vi "Dashboard Main.vi"() -> ()   [LabVIEW 2016]
uses:
  <vilib>/Utility/miscctls.llb/LVRowAndColumnTypeDef.ctl
  <vilib>/event_ctls.llb/eventvkey.ctl
  <vilib>/Rock Robotics/Network Tables/NT Write Boolean.vi
  <vilib>/Rock Robotics/Network Tables/NT Read Numeric Array.vi
  <vilib>/Rock Robotics/WPI/Dashboard/WPI_DashboardLogging Global.vi
  <vilib>/Utility/config.llb/Read Key (Double).vi
  <vilib>/Utility/config.llb/Write Key (Double).vi
  <vilib>/Utility/config.llb/NI_LVConfig.lvlib
panel:
  in  "Camera Settings Right":T1={"Frame Rate"=30, "Compression"=30, "Size"=1, "DB Camera Config"=FALSE} {"Frame Rate" scale=1.0..30.0; "Compression" scale=100.0..-1.0; "Size" items=["640x480", "320x240", "160x120"]}
  in  "Camera Name Right":string(combo)="No Camera Selection"
  out "Camera Info":cluster{"Mbps LED":bool, "Mbps":dbl, "fps":dbl} {"fps" format="%#.1g"; "Mbps" format="%#.1g"}
  in  "Camera Settings":T1={"Frame Rate"=30, "Compression"=30, "Size"=1, "DB Camera Config"=FALSE} {"Frame Rate" scale=1.0..30.0; "Compression" scale=100.0..-1.0; "Size" items=["640x480", "320x240", "160x120"]}
  in  "TCP":refnum<k5>
  in  "Rec Mode":enum32{"Stop", "Record", "Playback"}(radio)
  out "Robot IP":string
  out "Image Message":string="Timeout in Camera Communications"
  in  "Dashboard Tab":T2(tab)
  out "Gear Hopper State":string
  out "Ultrasonic Distance":dbl(slide) scale=0.0..5.0
  in  "Winch Reverse":bool
  in  "Enable PID":bool
  out "Drive Gear":string
  in  "Drive Mode":enum16{"Tank Drive", "Arcade Drive"}(ring)
  in  "Controller Mode":enum16{"X-Box Controller", "Joysticks"}(ring)
  out "Code Version":string
  out "Dashboard Version":string
  in  "Select Auto":string(combo)="Select Autonomous ..."
  out "NT Connection":bool
  out "MotorChart R":cluster{"Numeric":dbl, "Numeric":dbl}(graph)
  out "MotorChart L":cluster{"Numeric":dbl, "Numeric":dbl}(graph)
  out "MotorSliders R":cluster{"MotorSlide1":dbl, "MotorSlide2":dbl} {"MotorSlide2" scale=-1.0..1.0 scale format="%#_2e"; "MotorSlide1" scale=-1.0..1.0 scale format="%#_2e"}
  out "MotorSliders L":cluster{"MotorSlide1":dbl, "MotorSlide2":dbl} {"MotorSlide2" scale=-1.0..1.0 scale format="%#_2e"; "MotorSlide1" scale=-1.0..1.0 scale format="%#_2e"}
  out "Gyro":dbl(knob) scale=0.0..360.0
  out "JS1 Z":dbl(slide) scale=-1.0..1.0 scale format="%#_2e"
  out "JS1 Graph":cluster{"X":dbl, "Y":dbl}[](graph)
  out "JS1 Buttons":T3
  out "JS2 Z":dbl(slide) scale=-1.0..1.0 scale format="%#_2e"
  out "JS2 Graph":cluster{"X":dbl, "Y":dbl}[](graph)
  out "JS2 Buttons":T3
  out "Mode":T4(ring)=enum."Auto Disabled"
  out "Camera Image Right":T5(plugin-control)
  in  "DB/String 9":string
  in  "DB/String 8":string
  in  "DB/String 7":string
  in  "DB/String 6":string
  in  "DB/String 5":string
  in  "DB/String 4":string
  in  "DB/String 3":string
  in  "DB/String 2":string
  in  "DB/String 1":string
  in  "DB/String 0":string
  in  "DB/Slider 0":dbl(slide) scale=0.0..5.0
  in  "DB/Slider 1":dbl(slide) scale=0.0..5.0
  in  "DB/Slider 2":dbl(slide) scale=0.0..5.0
  in  "DB/Slider 3":dbl(slide) scale=0.0..5.0
  out "DB/LED 3":bool
  out "DB/LED 2":bool
  out "DB/LED 1":bool
  out "DB/LED 0":bool
  in  "DB/Button 3":bool
  in  "DB/Button 2":bool
  in  "DB/Button 1":bool
  in  "DB/Button 0":bool caption="New Name"
  in  "High Gear Multiplier":dbl(slide)=1.0 scale=0.0..1.0
  in  "Low Gear Multiplier":dbl(slide)=1.0 scale=0.0..1.0
  out "Robot Status":string
  in  "Ring Light Off":bool
  in  "Ring Light On":bool
  in  "Right Drive Bias":dbl(slide)=1.0 scale=0.9..1.0
  in  "Right Proportional Gain":dbl=0.02
  in  "Left Proportional Gain":dbl=0.02
  in  "Left Drive Bias":dbl(slide)=1.0 scale=0.9..1.0
  in  "Test Slider":dbl(slide) scale=0.0..100.0 scale format="%#_3g"
  in  "On/Off":bool caption="Solenoid"
  in  "Test Name":u16(ring) items=["Select the test to run..."]
  in  "Test Tree":string(tree)
  in  "Motor":cluster{"Value":dbl, "Enable":bool} {"Value" scale=-1.0..1.0 scale format="%#_3g"}
  out "Progress":T6 {"Test Progress" scale=0.0..100.0}
  in  "Rev/Fwd":cluster{"Forward":bool, "Reverse":bool}
  in  "Test Ring":u16(ring) items=["Monochrome", "Color"]
  out "Cmd Status":string
  in  "Execute Command":bool
  in  "Command Params":string[][](table)
  in  "Command Selection":i32(listbox)
  in  "CheckList":i32(listbox)
  out "Tree":string(tree)
  out "Camera Image":T5(plugin-control)
  out "Background":bool
  in  "Camera Name":string(combo)="No Camera Selection"
  # "HW"
  # "HW"
  # "Joysticks"
  # "Ultrasonic Distance"
  # "Drive Motors"
  # "Winch Reverse"
  # "Enable PID"
  # "Front"
  # "0.5"
  # "5"
  # "Controller Mode"
  # "Robot Code Version"
  # "Right"
  # "Left"
  # "Drive Mode"
  # "Dashboard Code Version"
  # "Back"
  # "This tab is a great place for autonomous settings and robot-specific values.\nPlace controls and indicators inside this tab and match name to\nDashboard Variables on robot. You can also delete this comment."
  # "Ring Light On"
  # "Left Drive Bias"
  # "Left Controller Gain"
  # "Right Controller Gain"
  # "Ring Light Off"
  # "Right Drive Bias"
  # "Robot Status"
  # "Low Gear Multiplier"
  # "High Gear Multiplier"
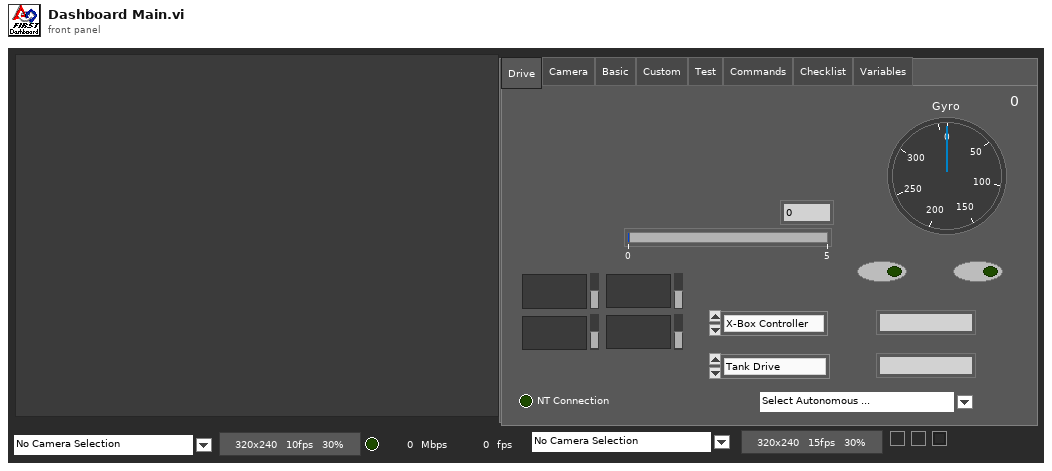
[diagram p1: front panel]
types:
  T1 = cluster{"Frame Rate":i32, "Compression":i32, "Size":u16, "DB Camera Config":bool}
  T2 = enum32{"Drive", "Camera", "Basic", "Custom", "Test", "Commands", "Checklist", "Variables"}
  T3 = cluster{bool, bool, bool, bool, bool, bool, bool, bool, bool, bool, bool, bool}
  T4 = enum8{"Tele-Op Disabled", "Tele-Op Enabled", "Auto Disabled", "Auto Enabled", "Test Disabled", "Test Enabled", "Disconnected", "No Code", "E-Stop"}
  T5 = typedef "IMAQ Image.ctl" = refnum<image>
  T6 = cluster{"Test Progress":u8, "Test Progress Text":string}
  T7 = typedef "Image Type" = u32
  T8 = cluster{"IDs":cluster{"RPC field ID":u16, "Unique ID":u16}, "String":string}
  T9 = enum32{"Drive", "Basic", "Custom", "Test", "Checklist", "Variables"}
  T10 = typedef "NI_LVConfig.lvlib/Config Data RefNum.ctl" = refnum<k1>
  T11 = cluster{"Camera Image":refnum<vi>, "Dashboard Tab":refnum<vi>, "Background":refnum<vi>, "Rec Mode":refnum<vi>, "Test Slider":refnum<vi>, "On/Off ":refnum<vi>, "Test Ring":refnum<vi>, "Rev/Fwd":refnum<vi>, "Test Name":refnum<vi>, "Motor":refnum<vi>, "Progress":refnum<vi>, "CheckList":refnum<vi>, "Tree":refnum<vi>, "Test Tree":refnum<vi>, "Command Params":refnum<vi>, "Command Selection":refnum<vi>, "Execute Command":refnum<vi>, "Cmd Status":refnum<vi>, "Camera Settings":refnum<vi>, "Camera Name":refnum<vi>, "Camera Info":refnum<vi>, "Camera Settings Right":refnum<vi>, "Camera Name Right":refnum<vi>, "Camera Image Right":refnum<vi>}
  T12 = cluster{"Measurement Parameter":i32, "Range Lower Value":dbl, "Range Upper Value":dbl, "Range":bool, "Measurement Type":bool}[]
  T13 = cluster{"Global Rectangle":cluster{"x1Left":i32, "y1Top":i32, "x2Right":i32, "y2Bottom":i32}, "Centroid":cluster{"x":sgl, "y":sgl}, "Object Size":u32, "Score":dbl}[]
  T14 = cluster{"Current Position":enum16{"Closed", "Open"}, "Current State":enum16{"Closed", "Shifting", "Open"}}
  T15 = cluster{"Current Gear":enum16{"Low", "High"}, "Gear Shift State":enum16{"Low", "Shifting", "High"}}
  T16 = cluster{"Error Strings":string, "Disable Counts":cluster{u16, u16}, "Rail Faults":cluster{u16, u16, u16}, "Robot IP":string, "DB Mode":u8, "Event Info":cluster{"Name":string, "Type":u8, "Number":u16, "Replay":u8}}
  T17 = cluster{"Storage":cluster{"Disk Free":u64, "RAM Block":u32, "RAM free":u32}, "CPU Utilization":cluster{"CPU % ISR":sgl, "CPU % Time Crit":sgl, "CPU % Timed Str":sgl, "CPU % High":sgl, "CPU % Above":sgl, "CPU % Normal":sgl, "CPU % Low":sgl}, "CAN":cluster{"% Bus Utilization":sgl, "Bus Off Cnt":u32, "TX_FIFO Full Cnt":u32, "Receive Error Cnt":u8, "Transmit Error Cnt":u8}, "HID":cluster{"HID Outputs":u32, "Rumble Low":u16, "Rumble High":u16}[]}
  T18 = cluster{"Status bits":cluster{"Test Mode":bool, "Autonomous":bool, "Enabled":bool, "Code Start":bool, "Brownout":bool, "Reserved 2":bool, "Reserved 3":bool, "E-Stop":bool}, "Code Trace":cluster{"Disabled":bool, "TeleOp":bool, "Auto":bool, "Test":bool}, "Controller Type":enum16{"unknown", "cRIO", "roboRio"}, "Code?":enum16{"unknown", "noCode", "code"}, "Battery V":dbl}
  T19 = cluster{"Control Bits":cluster{"TestMode":bool, "Autonomous":bool, "Enabled":bool, "FMS Present":bool, bool, bool, bool, "E-Stop":bool}, "Team Station ":u8, "Countdown":sgl, "Joystick Values":cluster{"Axes":dbl[], "Buttons":bool[], "POVs":i16[]}[]}
  T20 = cluster{"Axes":dbl[], "Buttons":bool[], "POVs":i16[]}[]
  T21 = cluster{"Axes":dbl[], "Buttons":bool[], "POVs":i16[]}
  T22 = cluster{"Buttons[0]":bool, "Buttons[1]":bool, "Buttons[2]":bool, "Buttons[3]":bool, "Buttons[4]":bool, "Buttons[5]":bool, "Buttons[6]":bool, "Buttons[7]":bool, "Buttons[8]":bool, "Buttons[9]":bool, "Buttons[10]":bool, "Buttons[11]":bool}
  T23 = cluster{"Operation":enum16{"Update", "Clear"}, "Color Box":u32}[]
  T24 = typedef "eventvkey.ctl" = enum16{"ASCII", "Enter", "Return", "Shift", "Ctrl", "Alt", "Cmd", "Opt", "Caps", "NumLock", "Clear", "Break", "Up", "Down", "Left", "Right", "Insert", "Delete", "Home", "End", "PageUp", "PageDown", "Escape", "Help", "Pause", "ScrollLock", "F1", "F2", "F3", "F4", "F5", "F6", "F7", "F8", "F9", "F10", "F11", "F12", "F13", "F14", "F15", "F16", "F17", "F18", "F19", "F20", "F21", "F22", "F23", "F24", "Play", "VolumeUp", "VolumeDown", "Mute", "Two Byte Char"}
  T25 = cluster{"Image Size":bool, "Image Type":bool, "Pixel Value":bool, "ROI Information":bool, "Zoom Factor":bool}
  T26 = cluster{"Operation":enum16{"Update", "Clear"}, "Color Box":u32}
  T27 = typedef "LVRowAndColumnTypeDef.ctl" = cluster{"Row":i32, "Column":i32}
  T28 = cluster{"Shift":bool, "Ctrl":bool, "Alt":bool, "Cmd":bool, "Opt":bool}
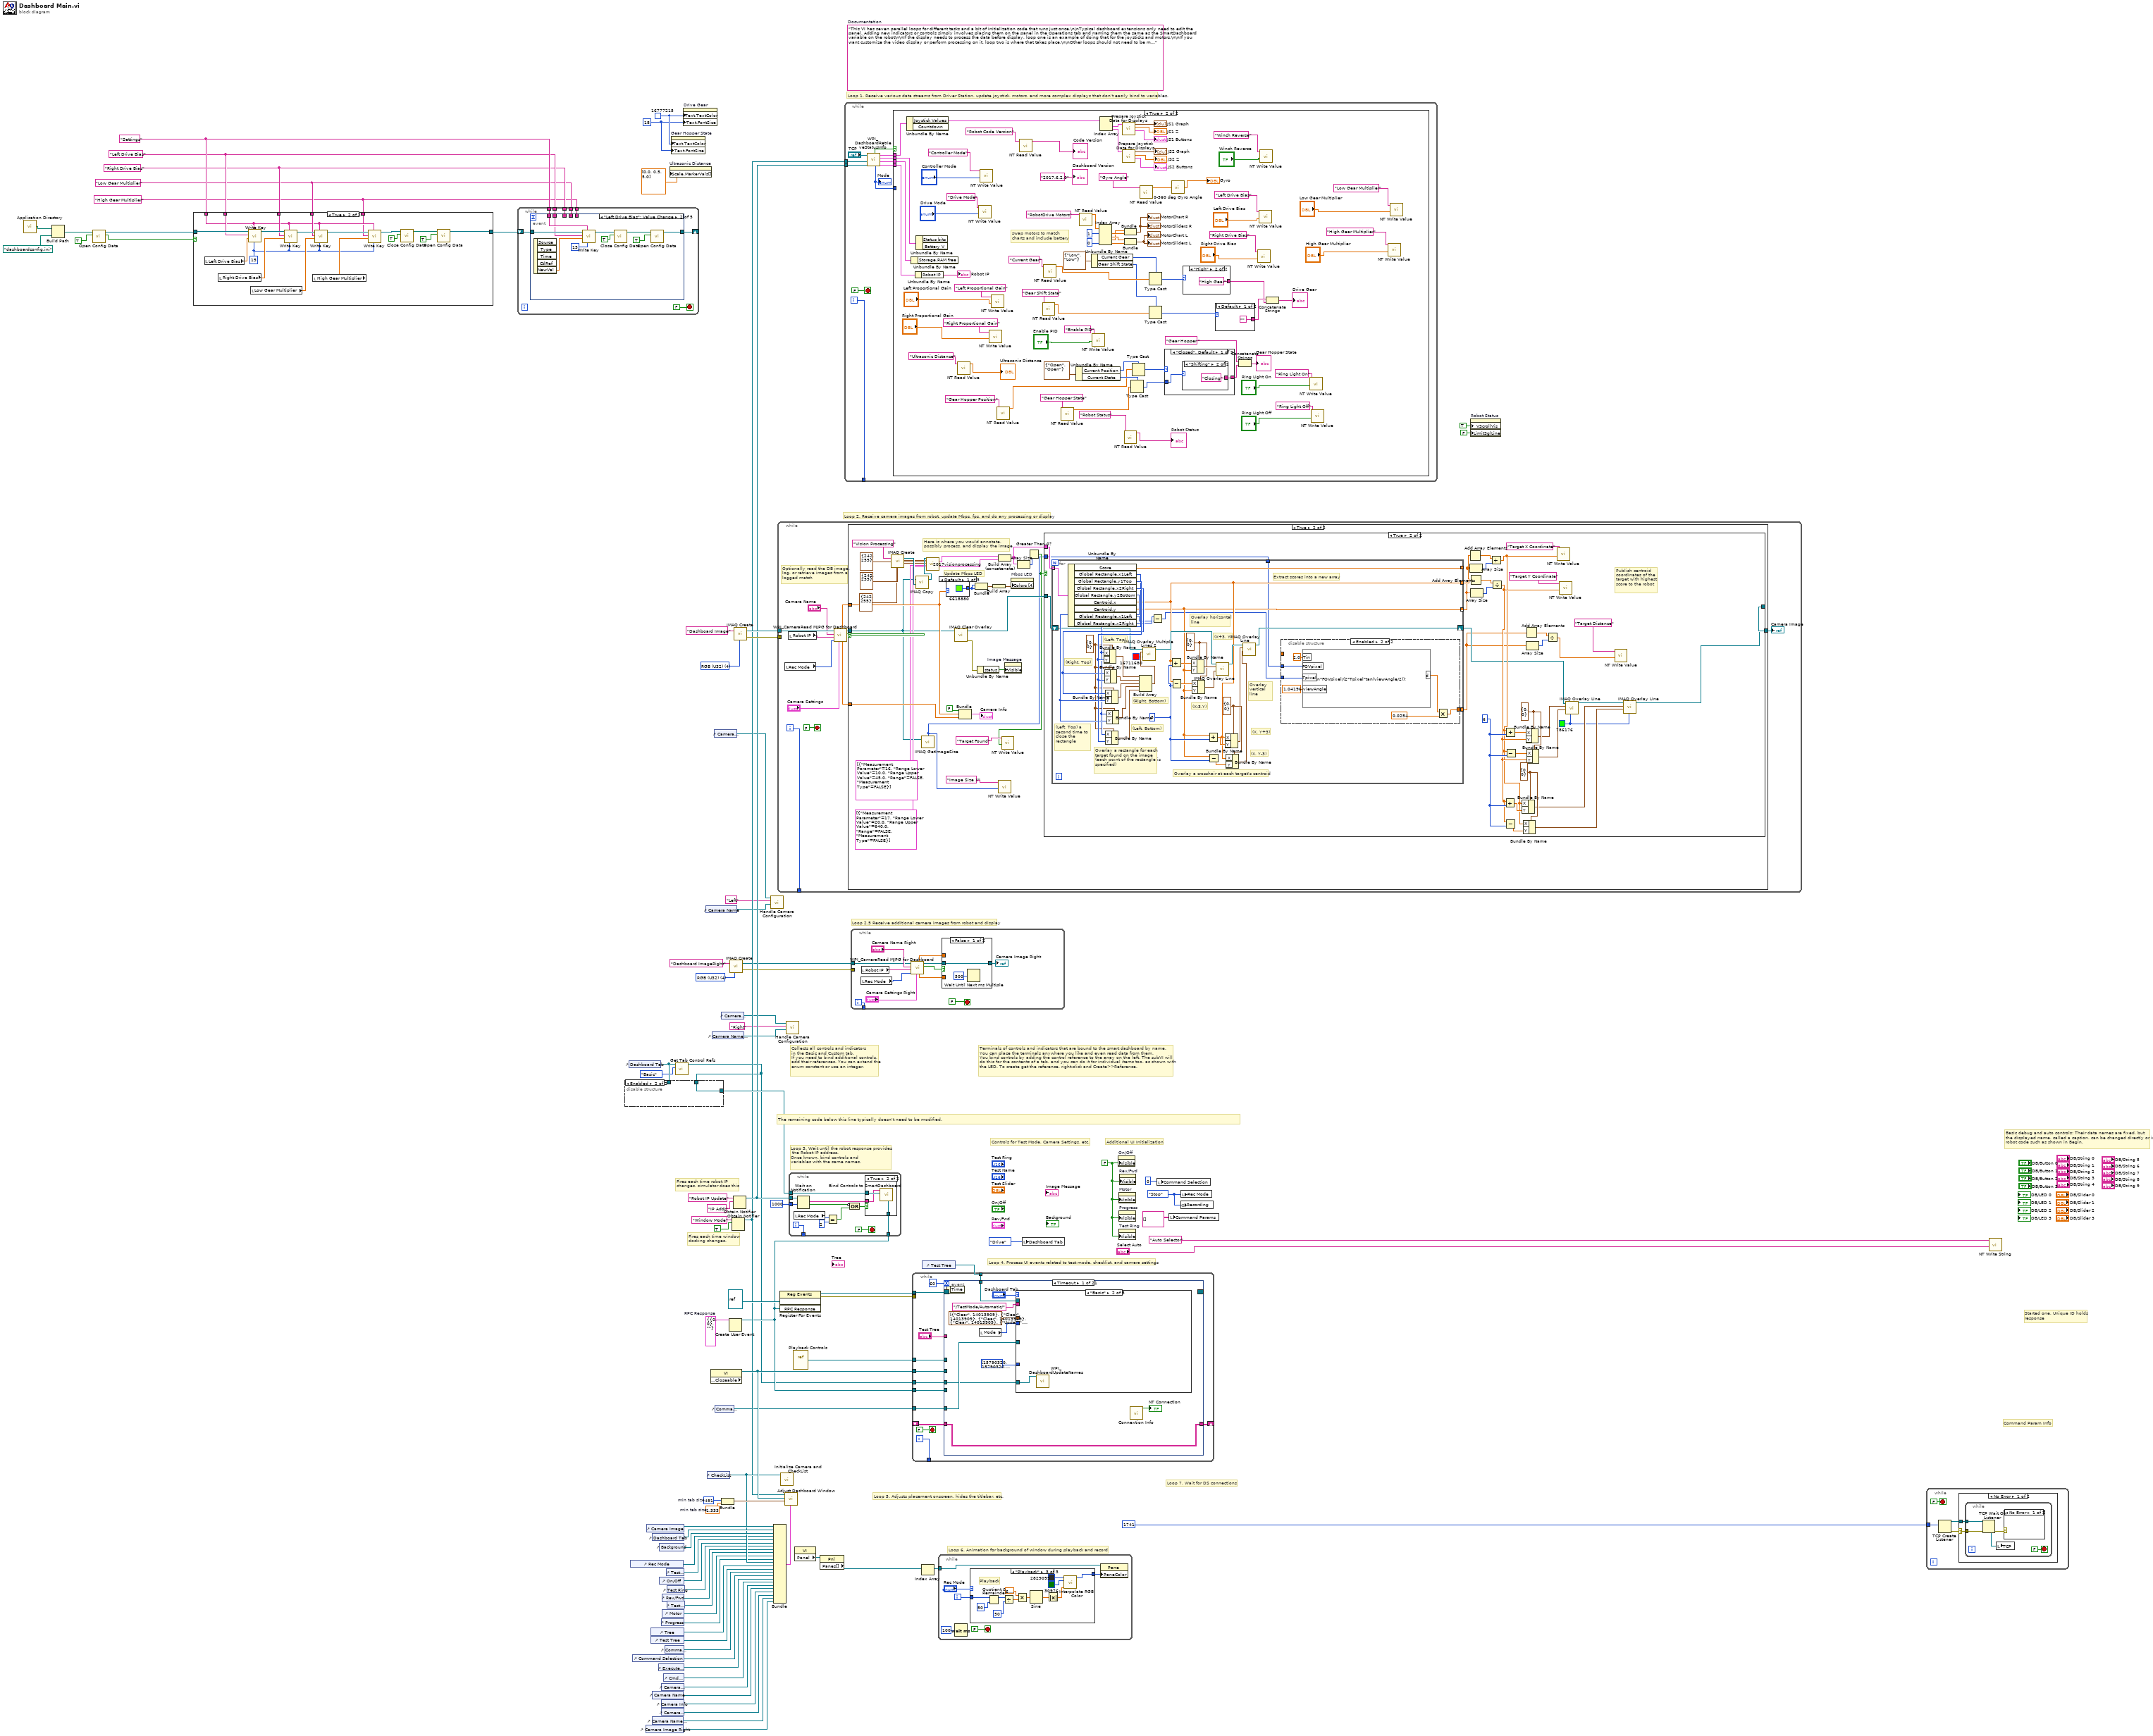
[diagram p0: block diagram]
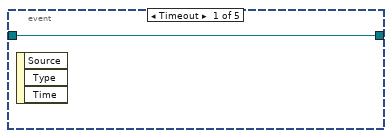
[diagram p2: hidden frame]
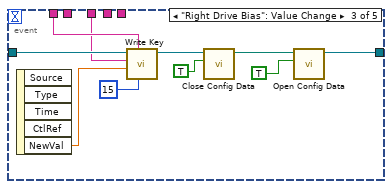
[diagram p3: hidden frame]
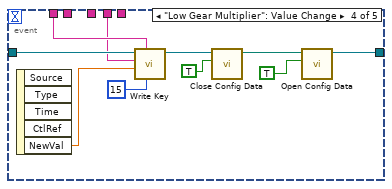
[diagram p4: hidden frame]
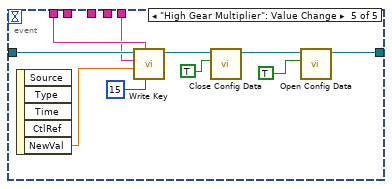
[diagram p5: hidden frame]
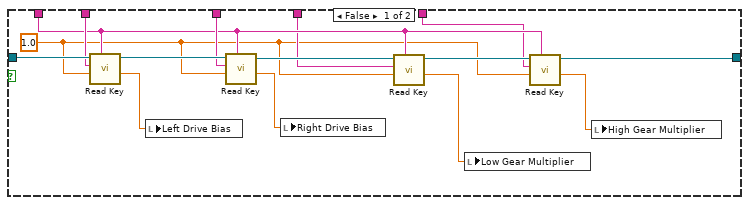
[diagram p6: hidden frame]
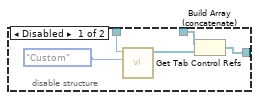
[diagram p7: hidden frame]
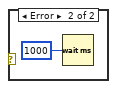
[diagram p9: hidden frame]
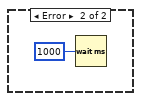
[diagram p10: hidden frame]
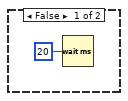
[diagram p11: hidden frame]
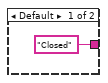
[diagram p12: hidden frame]
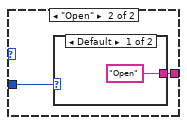
[diagram p13: hidden frame]
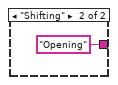
[diagram p14: hidden frame]
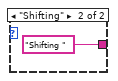
[diagram p15: hidden frame]
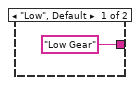
[diagram p16: hidden frame]
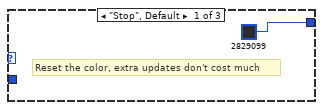
[diagram p17: hidden frame]
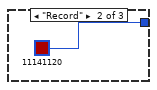
[diagram p18: hidden frame]
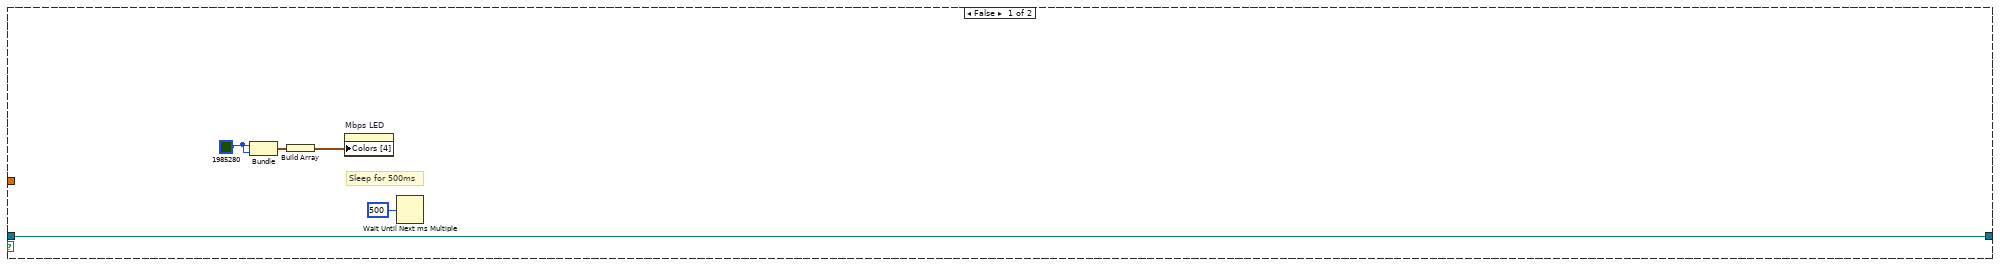
[diagram p20: hidden frame]
diagram:
  w1 = "High Gear Multiplier" ("Name")
  w2 = "Low Gear Multiplier" ("Name")
  w3 = u32 18 ("Text.Font:Size")
  w9 = "Right Drive Bias" ("Name")
  w10 = "Left Drive Bias" ("Name")
  w11 = "Settings"
  w6 = u32 16777215
  w27 = T7 4 items=["Grayscale (U8)", "Grayscale (I16)", "Grayscale (SGL)", "Complex (CSG)", "RGB (U32)", "HSL (U32)", "RGB (U64)"] ("Image Type")
  w43 = T8 {"IDs"={"RPC field ID"=0, "Unique ID"=0}, "String"=""}  # RPC Response
  w67 = 491  # min tab size
  w66 = 1.333  # min tab size
  w73 = enum32{"Stop", "Record", "Playback"}."Stop" ("Rec Mode")
  w50 = FALSE ("Visible")
  (unwired) "This VI has seven parallel loops for different tasks and a bit of initialization code that runs just once.\n\nTypical dashboard extensions only need to edit the panel. Adding new indicators or controls simply involves placing them on the panel in the Operations tab and naming them the same as the SmartDashboard variable on the robot\n\nIf the display needs to process the data before display, loop one is an example of doing that for the joysticks and motors.\n\nIf you want customize the video display or perform processing on it, loop two is where that takes place.\n\nOther loops should not need to be modified. They are pretty standard, and document the task they perform."  # Documentation
  w90 = T7 4 items=["Grayscale (U8)", "Grayscale (I16)", "Grayscale (SGL)", "Complex (CSG)", "RGB (U32)", "HSL (U32)", "RGB (U64)"] ("Image Type")
  # "Loop 2.5 Receive additional camera images from robot and display"
  # "Command Param Info"
  # "Started one, Unique ID holds\nresponse"
  # "Loop 7. Wait for DS connections"
  # "Basic debug and auto controls: Their data names are fixed, but\nthe displayed name, called a caption, can be changed directly or in\nrobot code such as shown in Begin."
  # "Controls for Test Mode, Camera Settings, etc."
  # "Additional UI Initialization"
  # "Loop 6. Animation for background of window during playback and record"
  # "Fires each time robot IP\nchanges, simulator does this"
  # "Fires each time window\ndocking changes."
  # "Collects all controls and indicators\nin the Basic and Custom tab.\nIf you need to bind additional controls,\nadd their references. You can extend the\nenum constant or use an integer."
  # "The remaining code below this line typically doesn't need to be modified."
  # "Loop 4. Process UI events related to test mode, checklist, and camera settings"
  # "Terminals of controls and indicators that are bound to the smart dashboard by name.\nYou can place the terminals anywhere you like and even read data from them.\nYou bind controls by adding the control reference to the array on the left. The subVI will\ndo this for the contents of a tab, and you can do it for individual items too, as shown with\nthe LED. To create get the reference, right-click and Create>>Reference."
  # "Loop 3. Wait until the robot response provides\n the Robot IP address.\nOnce known, bind controls and\nvariables with the same names."
  # "Loop 5. Adjusts placement onscreen, hides the titlebar, etc."
  # "Loop 1. Receive various data streams from Driver Station, update joystick, motors, and more complex displays that don't easily bind to variables."
  # "Loop 2. Receive camera images from robot, update Mbps, fps, and do any processing or display"
  n1 = call <vilib>:"Application Directory.vi"() -> ("Application Directory"=w8:path)
  n2 = Build Path(base path=w8, name or relative path=path "dashboardconfig.ini") -> (appended path=w15:path)
  n3 = call <vilib>:"Open Config Data.vi"("create file if necessary (T)"=TRUE, "configuration file path"=w15) -> ("file created?"=w14:bool, "refnum"=w13:T10)  [unwired: 7 in, 1 out]
  n4 = case shown="True" w14 {
    tunnel: w13 -> [w105 w124]
    tunnel: [w97 w119] -> w12
    tunnel: w11 -> [w96 w110]
    tunnel: w10 -> [w104 w116]
    tunnel: w9 -> [w102 w115]
    tunnel: w2 -> [w95 w112]
    tunnel: w1 -> [w94 w108]
    frame False {
      w93 = 1.0 ("default value")
      n5 = call-poly <vilib>:"Read Key.vi"("section"=w96, "default value"=w93, "key"=w104, "refnum"=w105) -> ("value"=w101:dbl, "refnum out"=w103:T10)  [unwired: 4 in, 2 out]
      n6 = local write "Left Drive Bias"(w101) -> ()
      n7 = call-poly <vilib>:"Read Key.vi"("section"=w96, "default value"=w93, "key"=w102, "refnum"=w103) -> ("value"=w100:dbl, "refnum out"=w99:T10)  [unwired: 4 in, 2 out]
      n8 = local write "Right Drive Bias"(w100) -> ()
      n9 = call-poly <vilib>:"Read Key.vi"("section"=w96, "default value"=w93, "key"=w95, "refnum"=w99) -> ("value"=w92:dbl, "refnum out"=w98:T10)  [unwired: 4 in, 2 out]
      n10 = local write "Low Gear Multiplier"(w92) -> ()
      n11 = call-poly <vilib>:"Read Key.vi"("section"=w96, "default value"=w93, "key"=w94, "refnum"=w98) -> ("value"=w91:dbl, "refnum out"=w97:T10)  [unwired: 4 in, 2 out]
      n12 = local write "High Gear Multiplier"(w91) -> ()
    }
    frame True {
      w106 = i16 15 ("precision (6)")
      n13 = local read "Left Drive Bias"() -> (w118:dbl)
      n14 = local read "Right Drive Bias"() -> (w117:dbl)
      n15 = call-poly <vilib>:"Write Key.vi"("precision (6)"=w106, "section"=w110, "value"=w118, "key"=w116, "refnum"=w124) -> ("refnum out"=w123:T10)  [unwired: 4 in, 2 out]
      n16 = local read "Low Gear Multiplier"() -> (w113:dbl)
      n17 = call-poly <vilib>:"Write Key.vi"("precision (6)"=w106, "section"=w110, "value"=w117, "key"=w115, "refnum"=w123) -> ("refnum out"=w114:T10)  [unwired: 4 in, 2 out]
      n18 = local read "High Gear Multiplier"() -> (w109:dbl)
      n19 = call-poly <vilib>:"Write Key.vi"("precision (6)"=w106, "section"=w110, "value"=w113, "key"=w112, "refnum"=w114) -> ("refnum out"=w111:T10)  [unwired: 4 in, 2 out]
      n20 = call-poly <vilib>:"Write Key.vi"("precision (6)"=w106, "section"=w110, "value"=w109, "key"=w108, "refnum"=w111) -> ("refnum out"=w107:T10)  [unwired: 4 in, 2 out]
      n21 = call <vilib>:"Close Config Data.vi"("write file if changed (T)"=TRUE, "refnum"=w107) -> ("file path"=w120:path)  [unwired: 8 in, 1 out]
      n22 = call <vilib>:"Open Config Data.vi"("create file if necessary (T)"=TRUE, "configuration file path"=w120) -> ("refnum"=w119:T10)  [unwired: 7 in, 2 out]
    }
  }
  n23 = while {
    shift-right: [w131] -> _
    shift-left: w12 -> [w130]
    tunnel: w11 -> [w129]
    tunnel: w10 -> [w128]
    tunnel: w9 -> [w127]
    tunnel: w2 -> [w126]
    tunnel: w1 -> [w125]
    stop <- FALSE stop-if-true
    n24 = event shown="[1] \"Left Drive Bias\": Value Change" {
      selector: _ -> [_ _ _ _ _]
      dyn-events: _ -> [_ _ _ _ _]
      timeout: _ -> [_ _ _ _ _]
      tunnel: [w133 w138 w148 w158 w168] -> w131
      tunnel: w130 -> [w133 w137 w147 w157 w167]
      tunnel: w129 -> [_ w135 w145 w156 w166]
      tunnel: w128 -> [_ w134 _ _ _]
      tunnel: w127 -> [_ _ w144 _ _]
      tunnel: w126 -> [_ _ _ w155 _]
      tunnel: w125 -> [_ _ _ _ w165]
      event Timeout {
        n25 = event-data() -> ()  [unwired: 1 in, 3 out]
      }
      event "Left Drive Bias": Value Change {
        n26 = event-data() -> ("NewVal"=w136:dbl)  [unwired: 1 in, 4 out]
        n27 = call-poly <vilib>:"Write Key.vi"("precision (6)"=i16 15, "section"=w135, "value"=w136, "key"=w134, "refnum"=w137) -> ("refnum out"=w142:T10)  [unwired: 4 in, 2 out]
        n28 = call <vilib>:"Close Config Data.vi"("write file if changed (T)"=TRUE, "refnum"=w142) -> ("file path"=w140:path)  [unwired: 8 in, 1 out]
        n29 = call <vilib>:"Open Config Data.vi"("create file if necessary (T)"=TRUE, "configuration file path"=w140) -> ("refnum"=w138:T10)  [unwired: 7 in, 2 out]
      }
      event "Right Drive Bias": Value Change {
        n30 = event-data() -> ("NewVal"=w146:dbl)  [unwired: 1 in, 4 out]
        n31 = call-poly <vilib>:"Write Key.vi"("precision (6)"=i16 15, "section"=w145, "value"=w146, "key"=w144, "refnum"=w147) -> ("refnum out"=w152:T10)  [unwired: 4 in, 2 out]
        n32 = call <vilib>:"Close Config Data.vi"("write file if changed (T)"=TRUE, "refnum"=w152) -> ("file path"=w150:path)  [unwired: 8 in, 1 out]
        n33 = call <vilib>:"Open Config Data.vi"("create file if necessary (T)"=TRUE, "configuration file path"=w150) -> ("refnum"=w148:T10)  [unwired: 7 in, 2 out]
      }
      event "Low Gear Multiplier": Value Change {
        n34 = event-data() -> ("NewVal"=w154:dbl)  [unwired: 1 in, 4 out]
        n35 = call-poly <vilib>:"Write Key.vi"("precision (6)"=i16 15, "section"=w156, "value"=w154, "key"=w155, "refnum"=w157) -> ("refnum out"=w162:T10)  [unwired: 4 in, 2 out]
        n36 = call <vilib>:"Close Config Data.vi"("write file if changed (T)"=TRUE, "refnum"=w162) -> ("file path"=w160:path)  [unwired: 8 in, 1 out]
        n37 = call <vilib>:"Open Config Data.vi"("create file if necessary (T)"=TRUE, "configuration file path"=w160) -> ("refnum"=w158:T10)  [unwired: 7 in, 2 out]
      }
      event "High Gear Multiplier": Value Change {
        n38 = event-data() -> ("NewVal"=w164:dbl)  [unwired: 1 in, 4 out]
        n39 = call-poly <vilib>:"Write Key.vi"("precision (6)"=i16 15, "section"=w166, "value"=w164, "key"=w165, "refnum"=w167) -> ("refnum out"=w172:T10)  [unwired: 4 in, 2 out]
        n40 = call <vilib>:"Close Config Data.vi"("write file if changed (T)"=TRUE, "refnum"=w172) -> ("file path"=w170:path)  [unwired: 8 in, 1 out]
        n41 = call <vilib>:"Open Config Data.vi"("create file if necessary (T)"=TRUE, "configuration file path"=w170) -> ("refnum"=w168:T10)  [unwired: 7 in, 2 out]
      }
    }
  }
  n42 = control-ref of="Dashboard Tab"() -> (w71:refnum<vi>)
  n43 = control-ref of="Rec Mode"() -> (w56:refnum<vi>)
  n44 = control-ref of="Command Selection"() -> (w42:refnum<vi>)
  n45 = control-ref of="Camera Image Right"() -> (w18:refnum<vi>)
  n46 = control-ref of="Camera Image"() -> (w69:refnum<vi>)
  n47 = control-ref of="Tree"() -> (w60:refnum<vi>)
  n48 = control-ref of="Test Tree"() -> (w59:refnum<vi>)
  n49 = control-ref of="Dashboard Tab"() -> (w68:refnum<vi>)
  n50 = control-ref of="Camera Name"() -> (w33:refnum<vi>)
  n51 = control-ref of="Camera Name Right"() -> (w19:refnum<vi>)
  n52 = control-ref of="Execute Command"() -> (w44:refnum<vi>)
  n53 = control-ref of="Background"() -> (w64:refnum<vi>)
  n54 = control-ref of="On/Off"() -> (w54:refnum<vi>)
  n55 = control-ref of="Progress"() -> (w51:refnum<vi>)
  n56 = control-ref of="Camera Settings"() -> (w34:refnum<vi>)
  n57 = control-ref of="Camera Info"() -> (w32:refnum<vi>)
  n58 = control-ref of="Camera Settings Right"() -> (w20:refnum<vi>)
  n59 = control-ref of="Rev/Fwd"() -> (w52:refnum<vi>)
  n60 = control-ref of="Motor"() -> (w57:refnum<vi>)
  n61 = control-ref of="Cmd Status"() -> (w38:refnum<vi>)
  n62 = control-ref of="Command Params"() -> (w45:refnum<vi>)
  n63 = control-ref of="Test Slider"() -> (w55:refnum<vi>)
  n64 = control-ref of="Test Ring"() -> (w53:refnum<vi>)
  n65 = control-ref of="Test Name"() -> (w58:refnum<vi>)
  n66 = property on="Ultrasonic Distance" class="Slide (strict)"("Scale.MarkerVals[]"=dbl[] [0.0, 0.5, 5.0] ("Scale.Marker Values[]")) -> ()  [unwired: 2 in, 2 out]
  n67 = property on="Gear Hopper State" class="Str"("Text.TextColor"=w6, "Text.FontSize"=w3) -> ()  [unwired: 2 in, 2 out]
  n68 = call <vilib>:"Get Tab Control Refs.vi"("Page Index"=T9."Basic" ("Dashboard Tab"), "TabControl in"=w71) -> ("ControlsOnPage"=w31:refnum<vi>[])  [unwired: 9 in]
  n69 = disable-structure shown="Enabled" {
    disable-tunnel: w71 -> [w178 _]
    disable-tunnel: [w176 w179] -> w70
    disable-tunnel: w31 -> [w174 w179]
    frame Disabled {
      n70 = call <vilib>:"Get Tab Control Refs.vi"("Page Index"=T9."Custom" ("Dashboard Tab"), "TabControl in"=w178) -> ("ControlsOnPage"=w177:refnum<vi>[])  [unwired: 9 in]
      n71 = Build Array (concatenate)(w174, w177) -> (w176:refnum<vi>[])
    }
    frame Enabled {
    }
  }
  n72 = property on="Drive Gear" class="Str"("Text.TextColor"=w6, "Text.FontSize"=w3) -> ()  [unwired: 2 in, 2 out]
  n73 = control-ref of="Camera Name"() -> (w35:refnum<vi>)
  n74 = control-ref of="CheckList"() -> (w61:refnum<vi>)
  n75 = property class="VI" props=["Front Panel.Closeable"]() -> (reference out=w72:refnum<vi>)  [unwired: 2 in, 2 out]
  n76 = control-ref of="Camera Name Right"() -> (w23:refnum<vi>)
  n77 = control-ref of="Camera Settings"() -> (w36:refnum<vi>)
  n78 = control-ref of="Command Params"() -> (w37:refnum<vi>)
  n79 = control-ref of="Camera Settings Right"() -> (w24:refnum<vi>)
  n80 = Bundle("min tab size"=w67, "min tab size"=w66) -> (w65:cluster{"min tab size":i32, "min tab size":dbl})  [unwired: 1 in]
  n81 = Create User Event(user event datatype=w43) -> (user event=w39:refnum<user-event>)  [unwired: 1 in, 1 out]
  n82 = call "IMAQ Create"("Image Name"="Dashboard ImageRight", "Image Type"=w27) -> ("New Image"=w26:T5, "error out"=w25:errorcluster)  [unwired: 2 in, 1 out]
  n83 = Obtain Notifier(name (unnamed)="Window Mode", notification data type=TRUE) -> (notifier out=w48:refnum<notifier>)  [unwired: 2 in, 2 out]
  n84 = Obtain Notifier(name (unnamed)="Robot IP Update", notification data type="IP Addr" ("name (unnamed)")) -> (notifier out=w49:refnum<notifier>)  [unwired: 2 in, 2 out]
  n85 = call "IMAQ Create"("Image Name"="Dashboard Image", "Image Type"=w90) -> ("New Image"=w88:T5, "error out"=w87:errorcluster)  [unwired: 2 in, 1 out]
  n86 = call "Handle Camera Configuration.vi"("CameraNameRef"=w35, "Camera File Name"="Left", "ClusterRef"=w36) -> ()  [unwired: 9 in]
  n87 = Bundle("Camera Image"=w69, "Dashboard Tab"=w68, "Background"=w64, "Rec Mode"=w56, "Test Slider"=w55, "On/Off"=w54, "Test Ring"=w53, "Rev/Fwd"=w52, "Test Name"=w58, "Motor"=w57, "Progress"=w51, "CheckList"=w61, "Tree"=w60, "Test Tree"=w59, "Command Params"=w45, "Command Selection"=w42, "Execute Command"=w44, "Cmd Status"=w38, "Camera Settings"=w34, "Camera Name"=w33, "Camera Info"=w32, "Camera Settings Right"=w20, "Camera Name Right"=w19, "Camera Image Right"=w18) -> (w62:T11)  [unwired: 1 in]
  n88 = while {
    tunnel: w88 -> [w189]
    tunnel: w87 -> [_]
    tunnel: [w190] -> _
    i -> [w190]
    stop <- FALSE stop-if-true
    # "Optionally read the DB image,\nlog, or retrieve images from a\nlogged match"
    n89 = local read "Rec Mode"() -> (w185:enum32{"Stop", "Record", "Playback"})
    n90 = local read "Robot IP"() -> (w184:string)
    n91 = call <vilib>:"WPI_CameraRead MJPG for Dashboard.vi"("Camera Settings"="Camera Settings", "Rec Mode"=w185, "Robot IP"=w184, "Camera Name"="Camera Name", "Refnum in"=w189) -> ("Active"=w187:bool, "Refnum out"=w188:T5, "FPS"=w186:dbl, "Bandwidth (Mbps)"=w183:dbl)  [unwired: 3 in]
    n92 = case shown="True" w187 {
      tunnel: w188 -> [w192 w201]
      tunnel: w183 -> [_ w218]
      tunnel: w186 -> [_ w219]
      tunnel: [w192 w214] -> w180
      frame False {
        w194 = u32 1985280 ("Color Box")
        # "Sleep for 500ms"
        n93 = Bundle("Color Box"=w194, "Color Box"=w194) -> (w195:cluster{"Color Box":u32, "Color Box":u32})  [unwired: 1 out]
        n94 = Build Array(w195) -> (w193:cluster{"Color Box":u32, "Color Box":u32}[])
        n95 = property on="Mbps LED" class="Bool (strict)"("Colors [4]"=w193) -> ()  [unwired: 2 in, 2 out]
        n96 = Wait Until Next ms Multiple(millisecond multiple=u32 500) -> ()  [unwired: 1 out]
      }
      frame True {
        # "Here is where you would annotate,\npossibly process, and display the image"
        # "Update Mbps LED"
        n97 = call "IMAQ Create"("Image Name"="Vision Processing") -> ("New Image"=w212:T5)  [unwired: 4 in, 1 out]
        n98 = call "IMAQ Copy"("Image Dst"=w212, "Image Src"=w201) -> ("Image Dst Out"=w211:T5)  [unwired: 4 in, 1 out]
        n99 = call "IMAQ GetImageSize"("Image"=w201) -> ("X Resolution"=w197:i32)  [unwired: 3 in, 2 out]
        n100 = call "2017visionprocessing.vi"("Image In"=w211, "Red or Hue Range (Color Threshold 1)"=cluster{"Lower value":i32, "Upper value":i32} {"Lower value"=242, "Upper value"=255}, "Green or Sat Range (Color Threshold 1)"=cluster{"Lower value":i32, "Upper value":i32} {"Lower value"=242, "Upper value"=255}, "Blue or Luma or Val or Inten Range (Color Threshold 1)"=cluster{"Lower value":i32, "Upper value":i32} {"Lower value"=242, "Upper value"=255}, "Selection Values (Particle Filter 1)"=T12 [{"Measurement Parameter"=16, "Range Lower Value"=10.0, "Range Upper Value"=45.0, "Range"=FALSE, "Measurement Type"=FALSE}], "Selection Values (Particle Filter 2)"=T12 [{"Measurement Parameter"=17, "Range Lower Value"=20.0, "Range Upper Value"=640.0, "Range"=FALSE, "Measurement Type"=FALSE}]) -> ("Shape Report (Shape Matching 1)"=w210:T13, "Shape Report (Shape Matching 2)"=w209:T13)  [unwired: 14 in, 6 out]
        n101 = case shown="Default" w218 {
          tunnel: [u32 6618880 ("Color Box") u32 16776722 ("Color Box") u32 16716800 ("Color Box")] -> w221
          frame Default {
          }
          frame 4, 5 {
          }
          frame 6.. {
          }
        }
        n102 = call "IMAQ Clear Overlay"("Image"=w201) -> ("error out"=w223:errorcluster, "Image Out"=w215:T5)  [unwired: 2 in, 7 out]
        n103 = Bundle(FALSE, "Bandwidth (Mbps)"=w218, "FPS"=w219) -> (→"Camera Info":cluster{bool, "Bandwidth (Mbps)":dbl, "FPS":dbl})  [unwired: 1 in]
        n104 = Bundle("Color Box"=w221, "Color Box"=w221) -> (w222:cluster{"Color Box":u32, "Color Box":u32})  [unwired: 1 out]
        n105 = Unbundle By Name(w223) -> ("status"=w224:bool)
        n106 = Build Array(w222) -> (w220:cluster{"Color Box":u32, "Color Box":u32}[])
        n107 = Build Array (concatenate)(w210, w209) -> (w208:T13)
        n108 = call-poly <vilib>:"NT Write Value.vi"("Numeric"=w197, "Name"="Image Size X") -> ()  [unwired: 9 in, 1 out]
        n109 = property on="Image Message" class="Str"("Visible"=w224) -> ()  [unwired: 2 in, 2 out]
        n110 = property on="Mbps LED" class="Bool (strict)"("Colors [4]"=w220) -> ()  [unwired: 2 in, 2 out]
        n111 = Array Size(array=w208) -> (size(s)=w207:i32)
        n112 = Greater Than 0?(x=w207) -> (x > 0?=w203:bool)
        n113 = call-poly <vilib>:"NT Write Value.vi"("Boolean"=w203, "Name"="Target Found") -> ()  [unwired: 9 in, 1 out]
        n114 = case shown="True" w203 {
          tunnel: w208 -> [_ w258]
          tunnel: w215 -> [w225 w255]
          tunnel: [w225 w233] -> w214
          tunnel: w197 -> [_ w228]
          frame False {
          }
          frame True {
            w232 = u32 786176 ("Color")
            w240 = cluster{"X":i32, "Y":i32} {"X"=0, "Y"=0} ("Point Coordinates")
            w244 = 6 ("Y")
            w241 = cluster{"X":i32, "Y":i32} {"X"=0, "Y"=0} ("Point Coordinates")
            # "Publish centroid coordinates of the target with highest score to the robot"
            n115 = for {
              tunnel: w258 -> [w294] mode=indexing
              tunnel: [w293] -> _ mode=indexing
              shift-right: [w272] -> w234
              shift-left: w255 -> [w280]
              tunnel: [w265] -> w252 mode=indexing
              tunnel: [w264] -> w249 mode=indexing
              tunnel: w228 -> [w261]
              tunnel: [w259] -> w227 mode=indexing
              w270 = cluster{"X":i32, "Y":i32} {"X"=0, "Y"=0} ("Point Coordinates")
              w271 = 3
              w276 = cluster{"X":i32, "Y":i32} {"X"=0, "Y"=0} ("Point Coordinates")
              w286 = cluster{"X":i32, "Y":i32} {"X"=0, "Y"=0} ("Point Coordinates")
              # "(X, Y-3)"
              # "(X, Y+3)"
              # "Overlay vertical line"
              # "(X+3, Y)"
              # "(X-3,Y)"
              # "Overlay horizontal line"
              # "Overlay a crosshair at each target's centroid"
              # "Extract scores into a new array"
              # "(Left, Top) a second time to close the rectangle"
              # "(Left, Bottom)"
              # "(Right, Bottom)"
              # "(Right, Top)"
              # "(Left, Top)"
              # "Overlay a rectangle for each target found on the image (each point of the rectangle is specified)"
              n116 = Unbundle By Name(w294) -> ("Score"=w293:dbl, "Global Rectangle.x1Left"=w287:i32, "Global Rectangle.y1Top"=w290:i32, "Global Rectangle.x2Right"=w288:i32, "Global Rectangle.y2Bottom"=w289:i32, "Centroid.x"=w265:sgl, "Centroid.y"=w264:sgl, "Global Rectangle.x1Left"=w262:i32, "Global Rectangle.x2Right"=w263:i32)
              n117 = Bundle By Name(cluster=w286, "X"=w287, "Y"=w290) -> (w292:cluster{"X":i32, "Y":i32})
              n118 = Bundle By Name(cluster=w286, "X"=w288, "Y"=w290) -> (w285:cluster{"X":i32, "Y":i32})
              n119 = Bundle By Name(cluster=w286, "X"=w288, "Y"=w289) -> (w284:cluster{"X":i32, "Y":i32})
              n120 = Bundle By Name(cluster=w286, "X"=w287, "Y"=w290) -> (w291:cluster{"X":i32, "Y":i32})
              n121 = Bundle By Name(cluster=w286, "X"=w287, "Y"=w289) -> (w283:cluster{"X":i32, "Y":i32})
              n122 = Build Array(w292, w285, w284, w283, w291) -> (w282:cluster{"X":i32, "Y":i32}[])
              n123 = call "IMAQ Overlay Multiple Lines 2"("Image"=w280, "Line End Points"=w282, "Color"=u32 16711680) -> ("Image Out"=w274:T5)  [unwired: 11 in, 1 out]
              n124 = Subtract(x=w263, y=w262) -> (x-y=w260:i32)
              n125 = Add(x=w265, y=w271) -> (x+y=w278:sgl)
              n126 = Subtract(x=w265, y=w271) -> (x-y=w277:sgl)
              n127 = Bundle By Name(cluster=w276, "X"=w278, "Y"=w264) -> (w279:cluster{"X":i32, "Y":i32})
              n128 = Bundle By Name(cluster=w276, "X"=w277, "Y"=w264) -> (w275:cluster{"X":i32, "Y":i32})
              n129 = Add(x=w264, y=w271) -> (x+y=w267:sgl)
              n130 = Subtract(x=w264, y=w271) -> (x-y=w266:sgl)
              n131 = call "IMAQ Overlay Line"("End Point"=w275, "Start Point"=w279, "Image"=w274) -> ("Image Out"=w273:T5)  [unwired: 7 in, 1 out]
              n132 = Bundle By Name(cluster=w270, "X"=w265, "Y"=w267) -> (w269:cluster{"X":i32, "Y":i32})
              n133 = Bundle By Name(cluster=w270, "X"=w265, "Y"=w266) -> (w268:cluster{"X":i32, "Y":i32})
              n134 = call "IMAQ Overlay Line"("End Point"=w268, "Start Point"=w269, "Image"=w273) -> ("Image Out"=w272:T5)  [unwired: 7 in, 1 out]
              n135 = disable-structure shown="Enabled" {
                disable-tunnel: _ -> [w297 _]
                disable-tunnel: [_ w302] -> w259
                disable-tunnel: w261 -> [_ w301]
                disable-tunnel: w260 -> [_ w298]
                frame Disabled {
                  n136 = expression code="320/(x*tan(1.04196/2))"(w297) -> (w295:dbl)
                  n137 = Multiply(x=w295, y=0.0254) -> ()  [unwired: 1 out]
                }
                frame Enabled {
                  n138 = formula code="d=Tin*FOVpixel/(2*Tpixel*tan(viewAngle/2));"("Tin"=2.0 ("input variable"), "FOVpixel"=w301, "Tpixel"=w298, "viewAngle"=1.04196 ("input variable")) -> ("d"=w303:dbl)
                  n139 = Multiply(x=w303, y=0.0254) -> (x*y=w302:dbl)
                }
              }
            }
            n140 = Add Array Elements(numeric array=w252) -> (sum=w254:sgl)
            n141 = Add Array Elements(numeric array=w249) -> (sum=w251:sgl)
            n142 = Array Size(array=w252) -> (size(s)=w253:i32)
            n143 = Array Size(array=w249) -> (size(s)=w250:i32)
            n144 = Divide(x=w254, y=w253) -> (x/y=w242:sgl)
            n145 = Divide(x=w251, y=w250) -> (x/y=w243:sgl)
            n146 = Add(x=w243, y=w244) -> (x+y=w246:sgl)
            n147 = Add(x=w242, y=w244) -> (x+y=w248:sgl)
            n148 = Subtract(x=w243, y=w244) -> (x-y=w245:sgl)
            n149 = Subtract(x=w242, y=w244) -> (x-y=w247:sgl)
            n150 = Bundle By Name(cluster=w240, "X"=w242, "Y"=w246) -> (w237:cluster{"X":i32, "Y":i32})
            n151 = Bundle By Name(cluster=w240, "X"=w242, "Y"=w245) -> (w236:cluster{"X":i32, "Y":i32})
            n152 = Add Array Elements(numeric array=w227) -> (sum=w231:dbl)
            n153 = Bundle By Name(cluster=w241, "X"=w248, "Y"=w243) -> (w239:cluster{"X":i32, "Y":i32})
            n154 = Array Size(array=w227) -> (size(s)=w230:i32)
            n155 = Bundle By Name(cluster=w241, "X"=w247, "Y"=w243) -> (w238:cluster{"X":i32, "Y":i32})
            n156 = Divide(x=w231, y=w230) -> (x/y=w226:dbl)
            n157 = call-poly <vilib>:"NT Write Value.vi"("Numeric"=w242, "Name"="Target X Coordinate") -> ()  [unwired: 9 in, 1 out]
            n158 = call-poly <vilib>:"NT Write Value.vi"("Numeric"=w243, "Name"="Target Y Coordinate") -> ()  [unwired: 9 in, 1 out]
            n159 = call "IMAQ Overlay Line"("Color"=w232, "End Point"=w238, "Start Point"=w239, "Image"=w234) -> ("Image Out"=w235:T5)  [unwired: 6 in, 1 out]
            n160 = call-poly <vilib>:"NT Write Value.vi"("Numeric"=w226, "Name"="Target Distance") -> ()  [unwired: 9 in, 1 out]
            n161 = call "IMAQ Overlay Line"("Color"=w232, "End Point"=w236, "Start Point"=w237, "Image"=w235) -> ("Image Out"=w233:T5)  [unwired: 6 in, 1 out]
          }
        }
      }
    }
    "Camera Image" <- w180
  }
  n162 = register-events(refnum<vi> refnum, w39) -> (reference out=w77:refnum<event-registration>, error out=w76:errorcluster)  [unwired: 2 in]
  n163 = call "Initialize Camera and CheckList.vi"("ListBox in"=w61) -> ()  [unwired: 11 in]
  n164 = call "Adjust Dashboard Window.vi"("Sizing Refnums"=w62, "Size Constraints"=w65, "VI"=w72, "WIn Mode"=w48) -> ()  [unwired: 8 in]
  n165 = call "Handle Camera Configuration.vi"("CameraNameRef"=w23, "Camera File Name"="Right", "ClusterRef"=w24) -> ()  [unwired: 9 in]
  n166 = while {
    tunnel: w70 -> [w319]
    tunnel: w49 -> [w317]
    tunnel: [w315] -> _
    tunnel: u32 1000 ("milliseconds to wait") -> [w314]
    tunnel: w39 -> [w308]
    i -> [w315]
    stop <- FALSE stop-if-true
    n167 = local read "Rec Mode"() -> (w310:enum32{"Stop", "Record", "Playback"})
    n168 = Wait on Notification(notifier=w317, timeout in ms (-1)=w314) -> (notification=w316:string, timed out?=w312:bool)  [unwired: 2 in, 2 out]
    n169 = Equal?(x=w310, y=u16 2 ("Rec Mode")) -> (x = y?=w311:bool)
    n170 = Compound Arithmetic op=OR(invert w312, w311) -> (w313:bool)
    n171 = case shown="True" w313 {
      tunnel: w319 -> [_ w322]
      tunnel: w316 -> [_ w321]
      tunnel: w308 -> [_ w320]
      frame False {
      }
      frame True {
        n172 = call <vilib>:"Bind Controls to SmartDashboard.vi"("RPC ref"=w320, "Bound Control Refs"=w322, "Server IP Address"=w321) -> ()  [unwired: 9 in]
      }
    }
  }
  n173 = vi-ref "Playback Controls.vi"() -> (w78:refnum<vi>)
  n174 = property class="VI"() -> ("Panel"=w80:refnum<vi>)  [unwired: 2 in, 2 out]
  n175 = property class="Pnl"(reference=w80) -> ("Panes[]"=w81:refnum<vi>[])  [unwired: 1 in, 2 out]
  n176 = while {
    tunnel: [w332] -> _
    tunnel: w49 -> [w326]
    tunnel: w48 -> [w323]
    i -> [w332]
    stop <- FALSE stop-if-true
    n177 = call <vilib>:"WPI_DashboardRetrieveStatusInfo.vi"("Binding Refnum"=w326, "Window Mode Notifier"=w323, "TCP Cnx"="TCP") -> ("Power and Errors"=w327:T16, "Robot Metrics"=w330:T17, "Status Info"=w331:T18, "Control Info"=w328:T19, "Robot Mode"=w325:T4, "Process?"=w329:bool)  [unwired: 3 in]
    "Mode" <- w325
    n178 = case shown="True" w329 {
      tunnel: w331 -> [_ w416]
      tunnel: w330 -> [_ w415]
      tunnel: w328 -> [_ w414]
      tunnel: w327 -> [_ w413]
      tunnel: w325 -> [_ _]
      frame False {
        n179 = Wait (ms)(milliseconds to wait=u32 20) -> ()  [unwired: 1 out]
      }
      frame True {
        # "swap motors to match\ncharts and include battery"
        n180 = Unbundle By Name(w414) -> ("Joystick Values"=w404:T20)  [unwired: 1 out]
        n181 = Unbundle By Name(w415) -> ()  [unwired: 1 out]
        n182 = Unbundle By Name(w413) -> ("Robot IP"=→"Robot IP":string)
        n183 = Unbundle By Name(w416) -> ()  [unwired: 2 out]
        n184 = call-poly <vilib>:"NT Read Value.vi"("Name"="Ultrasonic Distance") -> ("Numeric"=→"Ultrasonic Distance":dbl)  [unwired: 9 in, 1 out]
        n185 = call-poly <vilib>:"NT Write Value.vi"("Numeric"="Drive Mode", "Name"="Drive Mode") -> ()  [unwired: 9 in, 1 out]
        n186 = call-poly <vilib>:"NT Write Value.vi"("Numeric"="Controller Mode", "Name"="Controller Mode") -> ()  [unwired: 9 in, 1 out]
        n187 = call-poly <vilib>:"NT Write Value.vi"("Numeric"="Right Proportional Gain", "Name"="Right Proportional Gain") -> ()  [unwired: 9 in, 1 out]
        n188 = call-poly <vilib>:"NT Write Value.vi"("Numeric"="Left Proportional Gain", "Name"="Left Proportional Gain") -> ()  [unwired: 9 in, 1 out]
        n189 = call-poly <vilib>:"NT Read Value.vi"("Name"="Gear Hopper Position") -> ("Numeric"=w351:dbl)  [unwired: 9 in, 1 out]
        n190 = call-poly <vilib>:"NT Read Value.vi"("Name"="Robot Code Version") -> ("String"=→"Code Version":string)  [unwired: 9 in, 1 out]
        n191 = call-poly <vilib>:"NT Read Value.vi"("Name"="Gear Shift State") -> ("Numeric"=w382:dbl)  [unwired: 9 in, 1 out]
        n192 = call-poly <vilib>:"NT Read Value.vi"("Name"="Current Gear") -> ("Numeric"=w381:dbl)  [unwired: 9 in, 1 out]
        n193 = call-poly <vilib>:"NT Read Value.vi"("Name"="Gear Hopper State") -> ("Numeric"=w350:dbl)  [unwired: 9 in, 1 out]
        n194 = Unbundle By Name(T14 {"Current Position"=enum."Open", "Current State"=enum."Open"} ("y")) -> ("Current Position"=w355:enum16{"Closed", "Open"}, "Current State"=w354:enum16{"Closed", "Shifting", "Open"})
        n195 = call-poly <vilib>:"NT Read Value.vi"("Name"="RobotDrive Motors") -> ("Numeric Array"=w394:dbl[])  [unwired: 9 in, 1 out]
        n196 = Unbundle By Name(T15 {"Current Gear"=enum."Low", "Gear Shift State"=enum."Low"} ("Gear Shift Data")) -> ("Current Gear"=w380:enum16{"Low", "High"}, "Gear Shift State"=w379:enum16{"Low", "Shifting", "High"})
        n197 = call-poly <vilib>:"NT Write Value.vi"("Boolean"="Enable PID", "Name"="Enable PID") -> ()  [unwired: 9 in, 1 out]
        n198 = Index Array(array=w394, index #1=1, index #4=0) -> (element #1=w408:dbl, element #2=w409:dbl, element #3=w407:dbl, element #4=w412:dbl)  [unwired: 2 in]
        n199 = Index Array(array=w404) -> (element #1=w403:T21, element #2=w399:T21)  [unwired: 2 in]
        n200 = call "Prepare Joystick Data for Displays.vi"("Joystick Values"=w399) -> ("Buttons"=→"JS2 Buttons":T22, "Z Axis"=→"JS2 Z":dbl, "Cartesian Data"=→"JS2 Graph":cluster{"X axis":dbl, "X axis":dbl}[])  [unwired: 8 in]
        n201 = call "Prepare Joystick Data for Displays.vi"("Joystick Values"=w403) -> ("Buttons"=→"JS1 Buttons":T22, "Z Axis"=→"JS1 Z":dbl, "Cartesian Data"=→"JS1 Graph":cluster{"X axis":dbl, "X axis":dbl}[])  [unwired: 8 in]
        n202 = Bundle("Numeric"=w407, "Numeric"=w408) -> (→"MotorChart R" →"MotorSliders R":cluster{"Numeric":dbl, "Numeric":dbl})  [unwired: 1 in]
        n203 = Bundle("Numeric"=w409, "Numeric"=w412) -> (→"MotorChart L" →"MotorSliders L":cluster{"Numeric":dbl, "Numeric":dbl})  [unwired: 1 in]
        n204 = call-poly <vilib>:"NT Read Value.vi"("Name"="Robot Status") -> ("String"=→"Robot Status":string)  [unwired: 9 in, 1 out]
        n205 = Type Cast(type=w354, x=w350) -> (*(type *) &x=w348:enum16{"Closed", "Shifting", "Open"})
        n206 = Type Cast(type=w355, x=w351) -> (*(type *) &x=w349:enum16{"Closed", "Open"})
        n207 = call-poly <vilib>:"NT Read Value.vi"("Name"="Gyro Angle") -> ("Numeric"=w361:dbl)  [unwired: 9 in, 1 out]
        n208 = Type Cast(type=w380, x=w381) -> (*(type *) &x=w378:enum16{"Low", "High"})
        n209 = Type Cast(type=w379, x=w382) -> (*(type *) &x=w377:enum16{"Low", "Shifting", "High"})
        n210 = case shown="\"Closed\", Default" w349 {
          tunnel: w348 -> [w418 w422]
          tunnel: [w417 w421] -> w346
          frame "Closed", Default {
            n211 = case shown="\"Shifting\"" w418 {
              tunnel: ["Closed" "Closing"] -> w417
              frame Default {
              }
              frame "Shifting" {
              }
            }
          }
          frame "Open" {
            n212 = case shown="Default" w422 {
              tunnel: ["Open" "Opening"] -> w421
              frame Default {
              }
              frame "Shifting" {
              }
            }
          }
        }
        n213 = call "0-360 deg Gyro Angle.vi"("Raw Angle"=w361) -> ("0-360 deg Angle"=→"Gyro":dbl)
        n214 = case shown="\"High\"" w378 {
          tunnel: ["Low Gear" "High Gear"] -> w375
          frame "Low", Default {
          }
          frame "High" {
          }
        }
        n215 = case shown="Default" w377 {
          tunnel: ["" "Shifting "] -> w376
          frame Default {
          }
          frame "Shifting" {
          }
        }
        n216 = Concatenate Strings("Gear Hopper " ("string"), w346) -> (→"Gear Hopper State":string)
        n217 = call-poly <vilib>:"NT Write Value.vi"("Numeric"="Right Drive Bias", "Name"="Right Drive Bias") -> ()  [unwired: 9 in, 1 out]
        n218 = call-poly <vilib>:"NT Write Value.vi"("Numeric"="Left Drive Bias", "Name"="Left Drive Bias") -> ()  [unwired: 9 in, 1 out]
        n219 = call-poly <vilib>:"NT Write Value.vi"("Boolean"="Winch Reverse", "Name"="Winch Reverse") -> ()  [unwired: 9 in, 1 out]
        n220 = Concatenate Strings(w376, w375) -> (→"Drive Gear":string)
        n221 = call-poly <vilib>:"NT Write Value.vi"("Boolean"="Ring Light On", "Name"="Ring Light On") -> ()  [unwired: 9 in, 1 out]
        n222 = call-poly <vilib>:"NT Write Value.vi"("Boolean"="Ring Light Off", "Name"="Ring Light Off") -> ()  [unwired: 9 in, 1 out]
        n223 = call-poly <vilib>:"NT Write Value.vi"("Numeric"="High Gear Multiplier", "Name"="High Gear Multiplier") -> ()  [unwired: 9 in, 1 out]
        n224 = call-poly <vilib>:"NT Write Value.vi"("Numeric"="Low Gear Multiplier", "Name"="Low Gear Multiplier") -> ()  [unwired: 9 in, 1 out]
        "Dashboard Version" <- "2017.6.2.0" ("Dashboard Version")
      }
    }
  }
  n225 = while {
    tunnel: w26 -> [w439]
    tunnel: w25 -> [_]
    tunnel: [w433] -> _
    i -> [w433]
    stop <- FALSE stop-if-true
    n226 = local read "Rec Mode"() -> (w437:enum32{"Stop", "Record", "Playback"})
    n227 = local read "Robot IP"() -> (w438:string)
    n228 = call <vilib>:"WPI_CameraRead MJPG for Dashboard.vi"("Camera Settings"="Camera Settings Right", "Rec Mode"=w437, "Robot IP"=w438, "Camera Name"="Camera Name Right", "Refnum in"=w439) -> ("Active"=w432:bool, "Refnum out"=w435:T5, "FPS"=w430:dbl, "Bandwidth (Mbps)"=w431:dbl)  [unwired: 3 in]
    n229 = case shown="False" w432 {
      tunnel: w435 -> [w441 w443]
      tunnel: w431 -> [_ _]
      tunnel: w430 -> [_ _]
      tunnel: [w441 w443] -> w429
      frame False {
        n230 = Wait Until Next ms Multiple(millisecond multiple=u32 500) -> ()  [unwired: 1 out]
      }
      frame True {
      }
    }
    "Camera Image Right" <- w429
  }
  n231 = Index Array(array=w81) -> (element=w79:refnum<vi>)  [unwired: 1 in]
  n232 = control-ref of="Test Tree"() -> (w82:refnum<vi>)
  n233 = while {
    tunnel: [w453] -> _
    tunnel: w82 -> [w452]
    tunnel: w78 -> [w451]
    tunnel: w77 -> [w450]
    tunnel: w76 -> [_]
    tunnel: w72 -> [w449]
    tunnel: w39 -> [w448]
    tunnel: w37 -> [w447]
    shift-right: [w446] -> _
    shift-left: _ -> [w445]
    tunnel: w31 -> [w444]
    i -> [w453]
    stop <- FALSE stop-if-true
    n234 = event shown="[0] Timeout" {
      selector: w450 -> [_ _ _ _ _ _ _ _ _ _ _ _ _ _ _ _ _ _ _ _ _]
      dyn-events: [_ _ _ _ _ _ _ _ _ _ _ _ _ _ _ _ w709 _ _ _ _] -> _
      timeout: u32 60 ("milliseconds to wait") -> [_ _ _ _ _ _ _ _ _ _ _ _ _ _ _ _ _ _ _ _ _]
      tunnel: w452 -> [w465 _ _ _ _ _ _ _ _ _ _ _ _ _ _ _ _ _ _ _ _]
      tunnel: "Test Tree" -> [_ _ _ _ _ _ _ _ _ _ _ w676 w684 w686 w690 w698 _ _ _ _ _]
      tunnel: w451 -> [_ _ _ _ _ _ _ _ _ _ _ _ _ _ _ _ w711 _ w729 _ _]
      tunnel: w449 -> [_ _ _ _ _ _ _ _ _ _ _ _ _ _ _ _ w707 _ _ _ _]
      tunnel: w448 -> [_ _ _ _ _ _ _ _ _ _ _ _ _ _ _ _ w703 _ _ _ _]
      tunnel: w447 -> [w460 _ _ _ _ _ w627 _ _ _ _ _ _ _ _ _ _ _ _ _ _]
      tunnel: [w459 w504 w606 w611 w620 w624 w625 w634 w644 w651 w663 w675 w682 w685 w689 w697 w702 w724 w726 w730 w741] -> w446
      tunnel: w445 -> [w459 w504 w606 w611 w620 w624 w625 _ _ w651 w663 w675 w682 w685 w689 w697 w702 w724 w726 w730 w741]
      tunnel: w444 -> [w457 _ _ _ _ _ _ _ _ _ _ _ _ _ _ _ _ _ _ _ _]
      event Timeout {
        n235 = event-data() -> ()  [unwired: 1 in, 1 out]
        n236 = local read "Mode"() -> (w462:T4)
        n237 = case shown="\"Basic\"" "Dashboard Tab" {
          tunnel: w465 -> [_ _ w481 _ _]
          tunnel: "/TestMode/Automatic/" ("Name Pattern") -> [_ _ w480 _ _]
          tunnel: T23 [{"Operation"=enum."Clear", "Color Box"=14013909}, {"Operation"=enum."Clear", "Color Box"=14013909}, {"Operation"=enum."Clear", "Color Box"=14013909}, {"Operation"=enum."Clear", "Color Box"=14013909}, {"Operation"=enum."Update", "Color Box"=14013909}, {"Operation"=enum."Update", "Color Box"=16777215}, {"Operation"=enum."Clear", "Color Box"=14013909}, {"Operation"=enum."Clear", "Color Box"=14013909}, {"Operation"=enum."Clear", "Color Box"=14013909}] -> [_ _ w473 _ w497]
          tunnel: w462 -> [_ _ w472 _ w496]
          tunnel: u32[] [15790320, 15790320, 15790320, 15790320, 16777215, 16777215, 15790320, 15790320, 15790320] -> [_ _ _ _ w502]
          tunnel: w460 -> [_ _ _ _ w490]
          tunnel: w457 -> [_ w467 _ _ _]
          frame "Custom", Default {
          }
          frame "Basic" {
            n238 = call <vilib>:"WPI_DashboardUpdateNames.vi"("Controls on Tab"=w467) -> ()  [unwired: 11 in]
          }
          frame "Test" {
            w479 = -2 ("Active Item:Row Number")
            n239 = Index Array(array=w473, index=w472) -> (element=w474:T26)
            n240 = Unbundle(w474) -> ("Operation"=w475:enum16{"Update", "Clear"}, "Color Box"=w476:u32)
            n241 = call <vilib>:"NT Read String.vi"("Name"="/TestMode/TestName") -> ("String"=w470:string)  [unwired: 9 in, 1 out]
            n242 = call <vilib>:"NT Read and Format Entries as Tree.vi"("Operation"=w475, "Name Pattern"=w480, "Tree Refnum"=w481) -> ()  [unwired: 7 in, 2 out]
            n243 = case shown="\"\"" w470 {
              tunnel: "/TestMode/TestProgress" ("Name") -> [w483 _]
              tunnel: "/TestMode/TestProgressText" ("Name") -> [w482 _]
              frame Default {
                n244 = call <vilib>:"NT Read Number.vi"("Name"=w483) -> ("Numeric"=w484:dbl)  [unwired: 9 in, 1 out]
                n245 = call <vilib>:"NT Read String.vi"("Name"=w482) -> ("String"=w485:string)  [unwired: 9 in, 1 out]
                n246 = Bundle("Numeric"=w484, "String"=w485) -> (→"Progress":cluster{"Numeric":dbl, "String":string})  [unwired: 1 in]
              }
              frame "" {
                n247 = property on="Progress" class="Clust (strict)"("Visible"=FALSE) -> ()  [unwired: 2 in, 2 out]
                n248 = local write "Test Name"(u16 0) -> ()
              }
            }
            n249 = property on="Test Tree" class="Tree (strict)"("Active Item Row Number"=w479, "ActiveColNum"=w479, "CellBG"=w476, "Active Item Row Number"=-1 ("Active Item:Row Number"), "CellBG"=u32 5789784 ("Color Box")) -> ()  [unwired: 2 in, 2 out]
          }
          frame "Variables" {
            n250 = control-ref of="Tree"() -> (w489:refnum<vi>)
            n251 = call <vilib>:"NT Read and Format Entries as Tree.vi"("Tree Refnum"=w489) -> ()  [unwired: 9 in, 2 out]
          }
          frame "Commands" {
            w498 = u32 5789784 ("Color Box")
            w499 = T27 {"Row"=-1, "Column"=-2} ("Active Cell:Active Cell")
            w501 = T27 {"Row"=-2, "Column"=-2} ("Active Cell:Active Cell")
            n252 = Index Array(array=w502, index=w496) -> (element=w500:u32)
            n253 = Index Array(array=w497, index=w496) -> (element=w495:T26)
            n254 = Unbundle(w495) -> ("Operation"=w494:enum16{"Update", "Clear"})  [unwired: 1 out]
            n255 = local read "Command Selection"() -> (w493:i32)
            n256 = property on="Command Selection" class="MCListbox (strict)"("ActiveCell"=w501, "CellBG"=w500, "ActiveCell"=w499, "CellBG"=w498) -> ()  [unwired: 2 in, 2 out]
            n257 = call <vilib>:"WPI_DashboardUpdate RPC Info.vi"("Operation"=w494) -> ("update"=w492:bool, "commands"=w491:string[][])  [unwired: 9 in]
            n258 = property on="Command Selection" class="MCListbox (strict)"("ItemNames"=w491) -> ()  [unwired: 2 in, 2 out]
            n259 = property on="Command Params" class="Tbl (strict)"("Active Cell"=w501, "Cell BG Color"=w500, "Active Cell"=w499, "Cell BG Color"=w498) -> ()  [unwired: 2 in, 2 out]
            n260 = call <vilib>:"WPI_DashboardUpdate Command Params.vi"("Update"=w492, "NewVal"=w493, "Commands"=w491, "Param Tbl"=w490) -> ()  [unwired: 7 in, 1 out]
          }
        }
        n261 = call <vilib>:"Connextion Info.vi"() -> ("Connected"=→"NT Connection":bool)  [unwired: 10 in, 1 out]
      }
      event "Test Tree": Value Change {
        # "Show appropriate\ncontrols"
        n262 = event-data() -> ("CtlRef"=w507:refnum<vi>, "NewVal"=w505:string)  [unwired: 1 in]
        n263 = call <vilib>:"WPI_UtilitiesGetTreeIOName.vi"("NewVal"=w505, "TreeControl in"=w507) -> ("I/O Name"=w508:string)  [unwired: 9 in]
        n264 = case shown="\"Camera\"" w508 {
          selector: w508 -> [_ w515 _ w537 w546 _]
          tunnel: w505 -> [_ _ w534 w536 _ w553]
          tunnel: cluster{string[]}[] [{["640x480", "320x240", "160x120"]}, {["Auto", "Fixed indoor", "Fixed outdoor 1", "Fixed outdoor 2", "Fixed fluorescent 1", "Fixed fluorescent 2", "Hold current"]}, {["Auto", "Flicker-free 50 Hz", "Flicker-free 60 Hz", "Hold current"]}, {["None", "Prioritize frame rate", "Prioritize image quality"]}, {["Monochrome", "Color"]}] -> [_ _ _ _ _ w552]
          frame Default {
            w510 = FALSE ("Visible")
            w509 = FALSE ("Visible")
            n265 = property on="Motor" class="Clust (strict)"("Visible"=w509) -> ()  [unwired: 2 in, 2 out]
            n266 = property on="Test Ring" class="Ring (strict)"("Visible"=w509) -> ()  [unwired: 2 in, 2 out]
            n267 = property on="Rev/Fwd" class="Clust (strict)"("Visible"=w510) -> ()  [unwired: 2 in, 2 out]
            n268 = property on="On/Off" class="Bool (strict)"("Visible"=w510) -> ()  [unwired: 2 in, 2 out]
            n269 = property on="Test Slider" class="Slide (strict)"("Visible"=w510) -> ()  [unwired: 2 in, 2 out]
          }
          frame "Analog Out", "Motor", "PWM" {
            w516 = FALSE ("Visible")
            n270 = case shown="\"Analog Out\"" w515 {
              tunnel: [1.0 ("Value") -1.0 ("Value") 0.0 ("Value")] -> w514
              tunnel: [255.0 ("Value") 1.0 ("Value") 5.0 ("Value")] -> w513
              tunnel: [128.0 ("Value") 0.0 ("Value") 0.0 ("Value")] -> w512
              tunnel: [64.0 ("Value") 0.5 ("Value") 1.0 ("Value")] -> w511
              frame "PWM" {
              }
              frame "Motor", Default {
              }
              frame "Analog Out" {
              }
            }
            n271 = property on="Motor" class="Clust (strict)"("Visible"=TRUE) -> ()  [unwired: 2 in, 2 out]
            n272 = property on="Value" class="Slide (strict)"("Value"=w512, "Scale.Minimum"=w514, "Scale.Maximum"=w513, "Scale.Increment"=w511) -> ()  [unwired: 2 in, 2 out]
            n273 = property on="On/Off" class="Bool (strict)"("Visible"=w516) -> ()  [unwired: 2 in, 2 out]
            n274 = property on="Test Slider" class="Slide (strict)"("Visible"=w516) -> ()  [unwired: 2 in, 2 out]
            n275 = property on="Test Ring" class="Ring (strict)"("Visible"=w516) -> ()  [unwired: 2 in, 2 out]
            n276 = property on="Rev/Fwd" class="Clust (strict)"("Visible"=w516) -> ()  [unwired: 2 in, 2 out]
          }
          frame "Servo" {
            w532 = FALSE ("Visible")
            n277 = call <vilib>:"NT Read Number.vi"("Name"=w534) -> ("Numeric"=w533:dbl)  [unwired: 9 in, 1 out]
            n278 = property on="Test Slider" class="Slide (strict)"("Visible"=TRUE, "Scale.Maximum"=170.0 ("Scale.Range:Maximum")) -> ()  [unwired: 2 in, 2 out]
            n279 = local write "Test Slider"(w533) -> ()
            n280 = property on="Motor" class="Clust (strict)"("Visible"=w532) -> ()  [unwired: 2 in, 2 out]
            n281 = property on="Rev/Fwd" class="Clust (strict)"("Visible"=w532) -> ()  [unwired: 2 in, 2 out]
            n282 = property on="On/Off" class="Bool (strict)"("Visible"=w532) -> ()  [unwired: 2 in, 2 out]
            n283 = property on="Test Ring" class="Ring (strict)"("Visible"=w532) -> ()  [unwired: 2 in, 2 out]
          }
          frame "Relay", "Solenoid" {
            w535 = FALSE ("Visible")
            n284 = property on="Motor" class="Clust (strict)"("Visible"=w535) -> ()  [unwired: 2 in, 2 out]
            n285 = property on="Test Slider" class="Slide (strict)"("Visible"=w535) -> ()  [unwired: 2 in, 2 out]
            n286 = Search and Replace String(input string=w536, search string="/Value  **", replace string="/Direction") -> (result string=w542:string)  [unwired: 5 in, 3 out]
            n287 = property on="Test Ring" class="Ring (strict)"("Visible"=w535) -> ()  [unwired: 2 in, 2 out]
            n288 = call <vilib>:"NT Read String.vi"("Name"=w542) -> ("String"=w540:string)  [unwired: 9 in, 1 out]
            n289 = Equal?(x="Both directions", y=w540) -> (x = y?=w538:bool)
            n290 = Not(x=w538) -> (.not. x?=w539:bool)
            n291 = property on="Rev/Fwd" class="Clust (strict)"("Visible"=w538) -> ()  [unwired: 2 in, 2 out]
            n292 = property on="On/Off" class="Bool (strict)"("Visible"=w539, "Caption.Text"=w537) -> ()  [unwired: 2 in, 2 out]
          }
          frame "Compressor", "Digital Out" {
            w545 = FALSE ("Visible")
            # "Get direction and finish"
            n293 = property on="Motor" class="Clust (strict)"("Visible"=w545) -> ()  [unwired: 2 in, 2 out]
            n294 = property on="Test Slider" class="Slide (strict)"("Visible"=w545) -> ()  [unwired: 2 in, 2 out]
            n295 = property on="Test Ring" class="Ring (strict)"("Visible"=w545) -> ()  [unwired: 2 in, 2 out]
            n296 = property on="On/Off" class="Bool (strict)"("Visible"=TRUE, "Caption.Text"=w546) -> ()  [unwired: 2 in, 2 out]
            n297 = property on="Rev/Fwd" class="Clust (strict)"("Visible"=FALSE) -> ()  [unwired: 2 in, 2 out]
          }
          frame "Camera" {
            n298 = call <vilib>:"Get Last Path Segment.vi"("String in"=w553) -> ("String out"=w554:string)  [unwired: 10 in]
            n299 = property on="On/Off" class="Bool (strict)"("Visible"=FALSE) -> ()  [unwired: 2 in, 2 out]
            n300 = property on="Motor" class="Clust (strict)"("Visible"=FALSE) -> ()  [unwired: 2 in, 2 out]
            n301 = property on="Rev/Fwd" class="Clust (strict)"("Visible"=FALSE) -> ()  [unwired: 2 in, 2 out]
            n302 = case shown="\"White Balance  **\"" w554 {
              tunnel: w553 -> [w560 w569 w578 w587 w596 _ w602]
              tunnel: w552 -> [w558 w566 w575 w584 w593 _ _]
              frame "Size  **" {
                n303 = Index Array(array=w558) -> (element=w557:cluster{string[]})  [unwired: 1 in]
                n304 = call <vilib>:"NT Read String.vi"("Name"=w560) -> ("String"=w559:string)  [unwired: 9 in, 1 out]
                n305 = Unbundle(w557) -> (w555:string[])
                n306 = Match First String(2:w555, 3:w559) -> (0:w556:i32)  [unwired: 1 out]
                n307 = property on="Test Ring" class="Ring (strict)"("Value"=w556, "Strings []"=w555) -> ()  [unwired: 2 in, 2 out]
                n308 = property on="Test Ring" class="Ring (strict)"("Visible"=TRUE) -> ()  [unwired: 2 in, 2 out]
                n309 = property on="Test Slider" class="Slide (strict)"("Visible"=FALSE) -> ()  [unwired: 2 in, 2 out]
              }
              frame "White Balance  **" {
                n310 = Index Array(array=w566, index=1) -> (element=w567:cluster{string[]})
                n311 = call <vilib>:"NT Read String.vi"("Name"=w569) -> ("String"=w568:string)  [unwired: 9 in, 1 out]
                n312 = Unbundle(w567) -> (w564:string[])
                n313 = Match First String(2:w564, 3:w568) -> (0:w563:i32)  [unwired: 1 out]
                n314 = property on="Test Ring" class="Ring (strict)"("Value"=w563, "Strings []"=w564) -> ()  [unwired: 2 in, 2 out]
                n315 = property on="Test Ring" class="Ring (strict)"("Visible"=TRUE) -> ()  [unwired: 2 in, 2 out]
                n316 = property on="Test Slider" class="Slide (strict)"("Visible"=FALSE) -> ()  [unwired: 2 in, 2 out]
              }
              frame "Exposure  **" {
                n317 = Index Array(array=w575, index=2) -> (element=w576:cluster{string[]})
                n318 = call <vilib>:"NT Read String.vi"("Name"=w578) -> ("String"=w577:string)  [unwired: 9 in, 1 out]
                n319 = Unbundle(w576) -> (w572:string[])
                n320 = Match First String(2:w572, 3:w577) -> (0:w573:i32)  [unwired: 1 out]
                n321 = property on="Test Ring" class="Ring (strict)"("Value"=w573, "Strings []"=w572) -> ()  [unwired: 2 in, 2 out]
                n322 = property on="Test Ring" class="Ring (strict)"("Visible"=TRUE) -> ()  [unwired: 2 in, 2 out]
                n323 = property on="Test Slider" class="Slide (strict)"("Visible"=FALSE) -> ()  [unwired: 2 in, 2 out]
              }
              frame "Exposure Priority  **" {
                n324 = Index Array(array=w584, index=3) -> (element=w585:cluster{string[]})
                n325 = call <vilib>:"NT Read String.vi"("Name"=w587) -> ("String"=w586:string)  [unwired: 9 in, 1 out]
                n326 = Unbundle(w585) -> (w581:string[])
                n327 = Match First String(2:w581, 3:w586) -> (0:w582:i32)  [unwired: 1 out]
                n328 = property on="Test Ring" class="Ring (strict)"("Value"=w582, "Strings []"=w581) -> ()  [unwired: 2 in, 2 out]
                n329 = property on="Test Ring" class="Ring (strict)"("Visible"=TRUE) -> ()  [unwired: 2 in, 2 out]
                n330 = property on="Test Slider" class="Slide (strict)"("Visible"=FALSE) -> ()  [unwired: 2 in, 2 out]
              }
              frame "Color Enable  **" {
                n331 = Index Array(array=w593, index=4) -> (element=w594:cluster{string[]})
                n332 = call <vilib>:"NT Read String.vi"("Name"=w596) -> ("String"=w595:string)  [unwired: 9 in, 1 out]
                n333 = Unbundle(w594) -> (w590:string[])
                n334 = Match First String(2:w590, 3:w595) -> (0:w591:i32)  [unwired: 1 out]
                n335 = property on="Test Ring" class="Ring (strict)"("Value"=w591, "Strings []"=w590) -> ()  [unwired: 2 in, 2 out]
                n336 = property on="Test Ring" class="Ring (strict)"("Visible"=TRUE) -> ()  [unwired: 2 in, 2 out]
                n337 = property on="Test Slider" class="Slide (strict)"("Visible"=FALSE) -> ()  [unwired: 2 in, 2 out]
              }
              frame Default {
                n338 = property on="Test Ring" class="Ring (strict)"("Visible"=FALSE) -> ()  [unwired: 2 in, 2 out]
                n339 = property on="Test Slider" class="Slide (strict)"("Visible"=FALSE) -> ()  [unwired: 2 in, 2 out]
              }
              frame "Brightness  **", "Color Level  **", "Compression  **", "FPS  **", "Sharpness  **" {
                n340 = call <vilib>:"NT Read Number.vi"("Name"=w602) -> ("Numeric"=w601:dbl)  [unwired: 9 in, 1 out]
                n341 = local write "Test Slider"(w601) -> ()
                n342 = property on="Test Slider" class="Slide (strict)"("Visible"=TRUE, "Scale.Maximum"=100.0 ("Scale.Range:Maximum")) -> ()  [unwired: 2 in, 2 out]
                n343 = property on="Test Ring" class="Ring (strict)"("Visible"=FALSE) -> ()  [unwired: 2 in, 2 out]
              }
            }
          }
        }
        n344 = property on="Progress" class="Clust (strict)"("Visible"=FALSE) -> ()  [unwired: 2 in, 2 out]
      }
      event "Test Name": Mouse Enter {
        # "Populate the ring with the list of tests"
        n345 = event-data() -> ()  [unwired: 1 in, 1 out]
        n346 = call <vilib>:"NT Read String Array.vi"("Name"="/TestMode/TestList") -> ("String Array"=w610:string[])  [unwired: 9 in, 1 out]
        n347 = Build Array (concatenate)("Select the test to run...", w610) -> (w609:string[])
        n348 = property on="Test Name" class="Ring (strict)"("Strings []"=w609) -> ()  [unwired: 2 in, 2 out]
      }
      event "Test Name": Value Change {
        w612 = FALSE ("Visible")
        # "Tell the robot the test name to run"
        n349 = event-data() -> ("NewVal"=w616:u16)  [unwired: 1 in]
        n350 = property on="Test Name" class="Ring (strict)"() -> ("Strings []"=w617:string[])  [unwired: 2 in, 2 out]
        n351 = local write "Progress"(T6 {"Test Progress"=0, "Test Progress Text"=""} ("Progress")) -> ()
        n352 = Index Array(array=w617, index=w616) -> (element=w615:string)
        n353 = call <vilib>:"NT Write String.vi"("String"=w615, "Name"="/TestMode/TestName") -> ()  [unwired: 9 in, 1 out]
        n354 = property on="Progress" class="Clust (strict)"("Visible"=TRUE) -> ()  [unwired: 2 in, 2 out]
        n355 = property on="Motor" class="Clust (strict)"("Visible"=w612) -> ()  [unwired: 2 in, 2 out]
        n356 = property on="Test Slider" class="Slide (strict)"("Visible"=w612) -> ()  [unwired: 2 in, 2 out]
        n357 = property on="On/Off" class="Bool (strict)"("Visible"=w612) -> ()  [unwired: 2 in, 2 out]
        n358 = property on="Rev/Fwd" class="Clust (strict)"("Visible"=w612) -> ()  [unwired: 2 in, 2 out]
        n359 = property on="Test Ring" class="Ring (strict)"("Visible"=w612) -> ()  [unwired: 2 in, 2 out]
      }
      event "Select Auto": Mouse Enter {
        # "Populate the combo box with the list of autonomous options"
        n360 = event-data() -> ()  [unwired: 1 in, 1 out]
        n361 = call <vilib>:"NT Read String Array.vi"("Name"="Auto List") -> ("String Array"=w619:string[])  [unwired: 9 in, 1 out]
        n362 = property on="Select Auto" class="CmbBox"("Strings[]"=w619) -> ()  [unwired: 2 in, 2 out]
      }
      event "Select Auto": Value Change {
        # "User modified the Auto Selection. Write to NT variable so robot knows."
        n363 = event-data() -> ("NewVal"=w622:string)  [unwired: 1 in]
        n364 = call <vilib>:"NT Write String.vi"("String"=w622, "Name"="Auto Selector") -> ()  [unwired: 9 in, 1 out]
      }
      event "Command Selection": Value Change {
        # "Get the params and show in table"
        n365 = event-data() -> ("NewVal"=w628:i32)  [unwired: 1 in]
        n366 = property on="Command Selection" class="MCListbox (strict)"() -> ("ItemNames"=w626:string[][])  [unwired: 2 in, 2 out]
        n367 = call <vilib>:"WPI_DashboardUpdate Command Params.vi"("NewVal"=w628, "Commands"=w626, "Param Tbl"=w627) -> ()  [unwired: 8 in, 1 out]
      }
      event "Execute Command": Value Change {
        # "Started one, Unique ID holds\nresponse"
        n368 = event-data() -> ()  [unwired: 1 in, 1 out]
        n369 = property on="Command Selection" class="MCListbox (strict)"() -> ("ItemNames"=w639:string[][])  [unwired: 2 in, 2 out]
        n370 = Index Array(array=w639, index (row)="Command Selection", index (col)=0) -> (element=w637:string)
        n371 = call <vilib>:"Invoke Commands.vi"("Command Params"="Command Params", "Function Name"=w637) -> ("Params"=w633:u8, "Started"=w632:bool)  [unwired: 7 in, 1 out]
        n372 = Array Subset(array="Command Params", length (row)=w633) -> (w634:string[][])  [unwired: 3 in]
        n373 = Select(t="Executing" ("Cmd Status"), s=w632, f="" ("Cmd Status")) -> (s? t:f=→"Cmd Status":string)
      }
      event "Command Selection": Double Click {
        n374 = event-data() -> ("Row"=w647:i32)  [unwired: 1 in]
        n375 = property on="Command Selection" class="MCListbox (strict)"() -> ("ItemNames"=w650:string[][])  [unwired: 2 in, 2 out]
        n376 = local read "Command Params"() -> (w646:string[][])
        n377 = Index Array(array=w650, index (row)=w647, index (col)=0) -> (element=w648:string)
        n378 = call <vilib>:"Invoke Commands.vi"("Command Params"=w646, "Function Name"=w648) -> ("Params"=w645:u8, "Started"=w640:bool)  [unwired: 7 in, 1 out]
        n379 = Array Subset(array=w646, length (row)=w645) -> (w644:string[][])  [unwired: 3 in]
        n380 = Select(t="Executing" ("Cmd Status"), s=w640, f="" ("Cmd Status")) -> (s? t:f=w641:string)
        n381 = local write "Cmd Status"(w641) -> ()
      }
      event "CheckList": Double Click {
        # "Shift clears all"
        # "Update symbols on the listbox"
        n382 = event-data() -> ("PlatMods.Shift"=w652:bool, "Row"=w654:i32)  [unwired: 1 in]
        n383 = case shown="True" w652 {
          tunnel: w654 -> [w658 _]
          tunnel: 1 -> [w657 _]
          frame False {
            n384 = property on="CheckList" class="LstBox (strict)"() -> ("Item Symbols"=w656:i32[])  [unwired: 2 in, 2 out]
            n385 = Replace Array Subset(array=w656, new element=w657, index=w658) -> (w655:i32[])
            n386 = property on="CheckList" class="LstBox (strict)"("Item Symbols"=w655) -> ()  [unwired: 2 in, 2 out]
          }
          frame True {
            w659 = 0 ("Top Row")
            n387 = property on="CheckList" class="LstBox (strict)"() -> ("Number of Rows"=w661:u32)  [unwired: 2 in, 2 out]
            n388 = Initialize Array(0, w661) -> (w660:i32[])
            n389 = property on="CheckList" class="LstBox (strict)"("Top Row"=w659, "Value"=w659, "Item Symbols"=w660) -> ()  [unwired: 2 in, 2 out]
          }
        }
      }
      event "CheckList": Key Down {
        # "Update symbols on the listbox\nLeft and right keys check and uncheck"
        n390 = event-data() -> ("VKey"=w665:T24)  [unwired: 1 in]
        n391 = case shown="\"Left\", \"Right\"" w665 {
          selector: w665 -> [w670 _]
          tunnel: eventvkey."Left" ("VKey") -> [w668 _]
          frame "Left", "Right" {
            n392 = Equal?(x=w668, y=w670) -> (x = y?=w669:bool)
            n393 = Select(t=0, s=w669, f=1) -> (s? t:f=w671:i32)
            n394 = property on="CheckList" class="LstBox (strict)"() -> ("Item Symbols"=w674:i32[])  [unwired: 2 in, 2 out]
            n395 = Replace Array Subset(array=w674, new element=w671, index="CheckList") -> (w673:i32[])
            n396 = property on="CheckList" class="LstBox (strict)"("Item Symbols"=w673) -> ()  [unwired: 2 in, 2 out]
          }
          frame Default {
          }
        }
      }
      event "Motor.Enable": Value Change {
        # "When the test mode otor enable helper is set, update that\ntree row item's value"
        n397 = event-data() -> ("NewVal"=w680:bool)  [unwired: 1 in]
        n398 = Unbundle("Motor") -> ("Value"=w679:dbl)  [unwired: 1 out]
        n399 = Select(t=w679, s=w680, f=0.0) -> (s? t:f=w677:dbl)
        n400 = call <vilib>:"NT Write Number.vi"("Numeric"=w677, "Name"=w676) -> ()  [unwired: 9 in, 1 out]
      }
      event "Test Slider": Value Change {
        # "When the test mode slider helper is set, update that\ntree row item's value"
        n401 = event-data() -> ("NewVal"=w683:dbl)  [unwired: 1 in]
        n402 = call <vilib>:"NT Write Number.vi"("Numeric"=w683, "Name"=w684) -> ()  [unwired: 9 in, 1 out]
      }
      event "On/Off": Value Change {
        # "When the test mode on/off helper value is set, update that\ntree row item's value"
        n403 = event-data() -> ("NewVal"=w688:bool)  [unwired: 1 in]
        n404 = Boolean To (0,1)(Boolean=w688) -> (0, 1=w687:i16)
        n405 = call <vilib>:"NT Write Number.vi"("Numeric"=w687, "Name"=w686) -> ()  [unwired: 9 in, 1 out]
      }
      event "Rev/Fwd": Value Change {
        # "When the test mode helper value for relays is set, update that\ntree row item's value"
        n406 = event-data() -> ("NewVal.Forward"=w696:bool, "NewVal.Reverse"=w695:bool)  [unwired: 1 in]
        n407 = Boolean To (0,1)(Boolean=w696) -> (0, 1=w692:i16)
        n408 = Boolean To (0,1)(Boolean=w695) -> (0, 1=w694:i16)
        n409 = Negate(x=w694) -> (-x=w693:i16)
        n410 = Add(x=w692, y=w693) -> (x+y=w691:i16)
        n411 = call <vilib>:"NT Write Number.vi"("Numeric"=w691, "Name"=w690) -> ()  [unwired: 9 in, 1 out]
      }
      event "Test Ring": Value Change {
        # "When a test mode helper value is selected from the ring,\nset the tree item's variable to the string value"
        n412 = event-data() -> ("NewVal"=w700:u16)  [unwired: 1 in]
        n413 = property on="Test Ring" class="Ring (strict)"() -> ("Strings []"=w701:string[])  [unwired: 2 in, 2 out]
        n414 = Index Array(array=w701, index=w700) -> (element=w699:string)
        n415 = call <vilib>:"NT Write String.vi"("String"=w699, "Name"=w698) -> ()  [unwired: 9 in, 1 out]
      }
      event "Rec Mode": Value Change {
        # "Update globals for recording mode and path to read log from.\nClear when logging and let NetworkTables set path for vision to\nuse."
        n416 = event-data() -> ("NewVal"=w712:enum32{"Stop", "Record", "Playback"})  [unwired: 1 in]
        n417 = global write "WPI_DashboardLogging Global.vi" "Logging Filename"(path "") -> ()
        n418 = global write "WPI_DashboardLogging Global.vi" "Recording"(w712) -> ()
        n419 = case shown="\"Playback\"" w712 {
          tunnel: w711 -> [_ w714 w723]
          tunnel: [_ _ w722] -> w709
          tunnel: [_ _ w721] -> _
          tunnel: w707 -> [_ _ w719]
          tunnel: cluster{i32, i32} {-250, 170} -> [_ _ w718]
          tunnel: [_ _ T25 {"Image Size"=TRUE, "Image Type"=TRUE, "Pixel Value"=TRUE, "ROI Information"=TRUE, "Zoom Factor"=FALSE} ("Image Information Shown:All Elements")] -> w705
          tunnel: [_ _ TRUE ("Zoom Factor")] -> w704
          tunnel: w703 -> [_ _ w715]
          frame Default {
          }
          frame "Stop", "Record" {
            # "Place Window too"
            n420 = invoke class="VI" method="FP.Close"(reference=w714) -> (reference out=w713:refnum<vi>)  [unwired: 2 in, 2 out]
            n421 = invoke class="VI" method="Abort VI"(reference=w713) -> ()  [unwired: 2 in, 3 out]
          }
          frame "Playback" {
            n422 = call "Open Playback Panel.vi"("Offset"=w718, "DB VI Ref"=w719, "Playback in"=w723) -> ("Playback out"=w720:refnum<vi>)  [unwired: 8 in]
            n423 = register-events(w720, w715) -> (reference out=w722:refnum<event-registration>, error out=w721:errorcluster)  [unwired: 2 in]
          }
        }
        n424 = property on="Camera Image" class="ImageControl"("Image Information Shown"=w705, "Image Information Visible"=w704) -> ()  [unwired: 2 in, 2 out]
        n425 = call <vilib>:"WPI_DashboardNT Log FieldName Cache.vi"("Operation"=enum16{"Lookup/Add", "Index", "Clear"}."Clear") -> ()  [unwired: 8 in, 3 out]
      }
      event Panel Close {
        w725 = enum32{"Stop", "Record", "Playback"}."Stop" ("Rec Mode")
        # "Playback window has been closed, abort"
        n426 = event-data() -> ()  [unwired: 1 in, 4 out]
        n427 = local write "Rec Mode"(w725) -> ()
        n428 = global write "WPI_DashboardLogging Global.vi" "Recording"(w725) -> ()
      }
      event Panel Close {
        # "Abort playback window and ourself"
        n429 = event-data() -> ()  [unwired: 1 in, 4 out]
        n430 = invoke class="VI" method="FP.Close"(reference=w729) -> (reference out=w728:refnum<vi>)  [unwired: 2 in, 2 out]
        n431 = invoke class="VI" method="Abort VI"(reference=w728) -> (error out=w727:errorcluster)  [unwired: 2 in, 2 out]
        n432 = invoke class="VI" method="Abort VI"(error in=w727) -> ()  [unwired: 2 in, 3 out]
      }
      event User Event {
        n433 = event-data() -> ("IDs"=w736:cluster{"RPC field ID":u16, "Unique ID":u16}, "String"=w735:string)  [unwired: 1 in]
        n434 = Bundle("IDs"=w736, "String"=w735) -> (w734:T8)  [unwired: 1 in]
        n435 = call <vilib>:"Retrieve RPC Response.vi"("RPC Response"=w734) -> ("Output"=w732:string[][])  [unwired: 10 in]
        n436 = Build Array (concatenate)(w730, w732) -> (w731:string[][])
        n437 = local write "Command Params"(w731) -> ()
        n438 = local write "Cmd Status"("" ("Cmd Status")) -> ()
      }
      event "Tree": Double Click {
        n439 = event-data() -> ("PlatMods"=w740:T28, "Tag"=w739:string)  [unwired: 1 in]
        n440 = Unbundle(w740) -> ("Shift"=w738:bool)  [unwired: 4 out]
        n441 = Not(x=w738) -> (.not. x?=w737:bool)
        n442 = call <vilib>:"NT Update Persistence.vi"("Persistence"=w737, "Name"=w739) -> ()  [unwired: 9 in, 1 out]
      }
    }
  }
  n443 = while {
    tunnel: w79 -> [w743]
    i -> [w746]
    stop <- FALSE stop-if-true
    n444 = Wait (ms)(milliseconds to wait=u32 100) -> ()  [unwired: 1 out]
    n445 = case shown="\"Playback\"" "Rec Mode" {
      tunnel: w746 -> [_ _ w761]
      tunnel: [u32 2829099 ("Base Color") u32 11141120 ("Target Color") w750] -> w742
      frame "Stop", Default {
        # "Reset the color, extra updates don't cost much"
      }
      frame "Record" {
      }
      frame "Playback" {
        # "Playback"
        n446 = Quotient & Remainder(x=w761, y=u32 50 ("milliseconds to wait")) -> (x-y*floor(x/y)=w757:u32)  [unwired: 1 out]
        n447 = Divide(x=w757, y=u32 50 ("milliseconds to wait")) -> (x/y=w754:dbl)
        n448 = Multiply(x=6.283185307179586, y=w754) -> (x*y=w759:dbl)
        n449 = Sine(x=w759) -> (sin(x)=w758:dbl)
        n450 = Absolute Value(x=w758) -> (abs(x)=w751:dbl)
        n451 = call "Interpolate RGB Color.vi"("Proportion"=w751, "Target Color"=u32 30976, "Base Color"=u32 2829099) -> ("Result Color"=w750:u32)  [unwired: 8 in]
      }
    }
    n452 = property class="Pane"(reference=w743, "PaneColor"=w742) -> ()  [unwired: 1 in, 2 out]
  }
  n453 = local write "Dashboard Tab"(T2."Drive" ("Dashboard Tab")) -> ()
  n454 = property on="On/Off" class="Bool (strict)"("Visible"=w50) -> ()  [unwired: 2 in, 2 out]
  n455 = property on="Motor" class="Clust (strict)"("Visible"=w50) -> ()  [unwired: 2 in, 2 out]
  n456 = property on="Progress" class="Clust (strict)"("Visible"=w50) -> ()  [unwired: 2 in, 2 out]
  n457 = property on="Test Ring" class="Ring (strict)"("Visible"=w50) -> ()  [unwired: 2 in, 2 out]
  n458 = property on="Rev/Fwd" class="Clust (strict)"("Visible"=w50) -> ()  [unwired: 2 in, 2 out]
  n459 = local write "Command Selection"(u16 0 ("milliseconds to wait")) -> ()
  n460 = local write "Command Params"(string[][] [] ("Command Params")) -> ()
  n461 = global write "WPI_DashboardLogging Global.vi" "Recording"(w73) -> ()
  n462 = local write "Rec Mode"(w73) -> ()
  n463 = property on="Robot Status" class="Str"("VScrollVis"=TRUE ("Vertical Scrollbar Visible"), "LimitSglLine"=FALSE ("Limit To Single Line?")) -> ()  [unwired: 2 in, 2 out]
  n464 = while {
    tunnel: u16 1741 ("timeout ms (25000)") -> [w763]
    stop <- FALSE stop-if-true
    n465 = TCP Create Listener(10:w763) -> (0:w762:errorcluster, 3:w764:refnum<k5>)  [unwired: 4 in, 1 out]
    n466 = case shown="No Error" w762 {
      selector: w762 -> [w766 _]
      tunnel: w764 -> [w767 _]
      frame No Error {
        n467 = while {
          tunnel: w767 -> [w770]
          tunnel: w766 -> [w769]
          stop <- FALSE stop-if-true
          n468 = TCP Wait On Listener(8:w769, 11:w770) -> (0:w771:errorcluster, 4:w772:refnum<k5>)  [unwired: 2 in, 3 out]
          n469 = local write "TCP"(w772) -> ()
          n470 = case shown="No Error" w771 {
            frame No Error {
            }
            frame Error {
              n471 = Wait (ms)(milliseconds to wait=u32 1000) -> ()  [unwired: 1 out]
            }
          }
        }
      }
      frame Error {
        n472 = Wait (ms)(milliseconds to wait=u32 1000) -> ()  [unwired: 1 out]
      }
    }
  }
  n473 = call <vilib>:"NT Write String.vi"("String"="Select Auto", "Name"="Auto Selector") -> ()  [unwired: 9 in, 1 out]
